vi "RIB - Fuse.vi"(0 "Limits File Path":path, 5 "Results File Path":path, 11 "error in":errorcluster) -> (4 "Results Data Array":string[][](array[string]), 15 "error out":errorcluster)   [LabVIEW 2024]
doc: "Template test"
uses:
  <vilib>/addons/_JKI Toolkits/State Machine/_JKI_lib_State_Machine.llb/Select State(s)_err__jki_lib_state_machine.vi
  <vilib>/addons/_JKI Toolkits/State Machine/_JKI_lib_State_Machine.llb/Select State(s)_bool__jki_lib_state_machine.vi
  <vilib>/addons/_JKI Toolkits/State Machine/_JKI_lib_State_Machine.llb/Periodic Trigger__ogtk__JKI-SM__jki_lib_state_machine.vi
  <userlib>/_OpenG.lib/file/file.llb/Strip Path Extension - String__ogtk.vi
  <vilib>/Utility/file.llb/Read Delimited Spreadsheet (string).vi
  <userlib>/_OpenG.lib/file/file.llb/openg_file.lvlib
  <userlib>/_OpenG.lib/appcontrol/appcontrol.llb/openg_application_control.lvlib
  <userlib>/_OpenG.lib/time/time.llb/openg_time.lvlib
  <vilib>/Utility/file.llb/Write Delimited Spreadsheet (string).vi
panel:
  in  "All Fuses Test":string
  in  "Fuse 9 Test":string
  in  "Fuse 8 Test":string
  in  "Fuse 7 Test":string
  in  "Fuse 6 Test":string
  in  "Fuse 5 Test":string
  in  "Fuse 4 Test":string
  in  "Fuse 3 Test":string
  out "All Fuses Test":bool
  out "Fuse 9 Test":bool
  out "Fuse 8 Test":bool
  out "Fuse 7 Test":bool
  out "Fuse 6 Test":bool
  out "Fuse 5 Test":bool
  out "Fuse 4 Test":bool
  out "Fuse 3 Test":bool
  out "Fuse 2 Test":bool
  out "Fuse 1 Test":bool
  in  "Fuse 2 Test":string
  in  "Fuse 1 Test":string
  in  "connection ID":refnum<k16>
  in  "handle out":u64
  in  "Exit":bool
  # "Fuse Test"
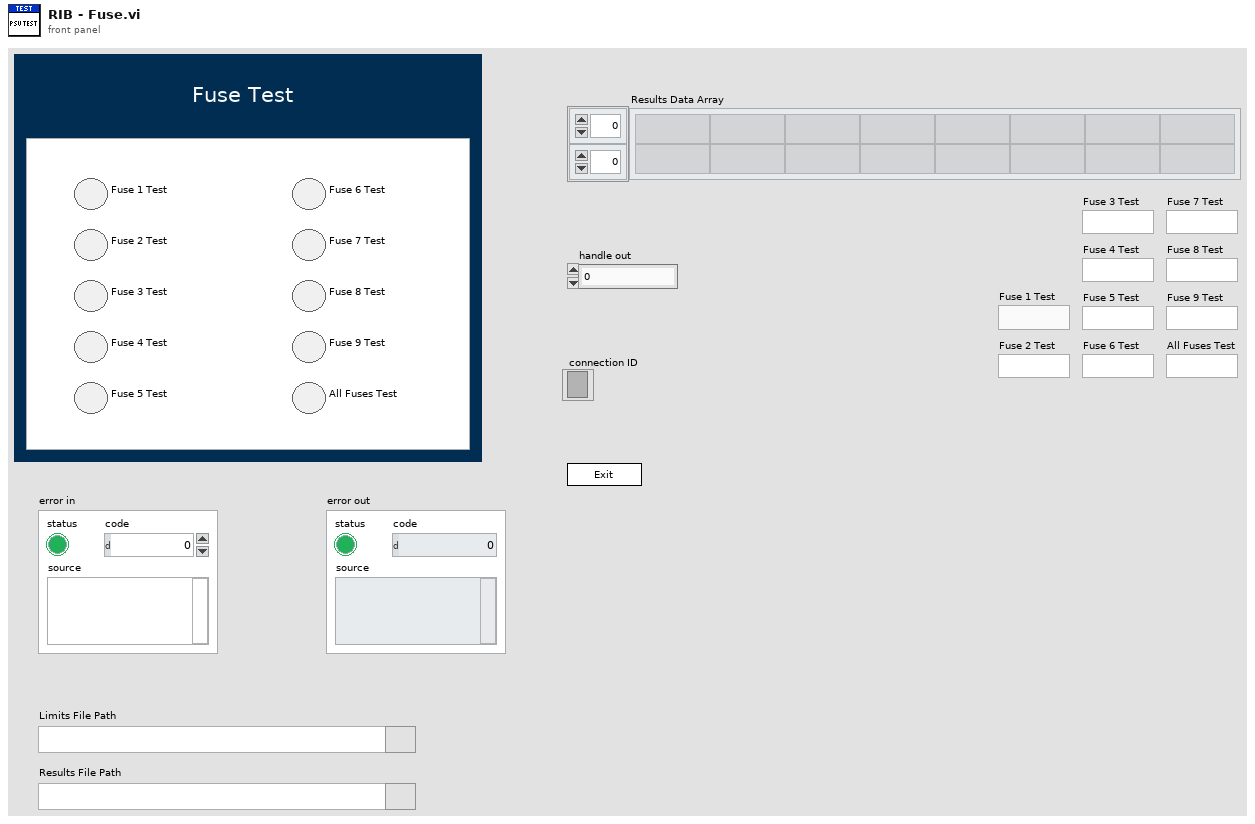
[diagram p1: front panel]
types:
  T1 = enum32{"Invalid", "Standard", "Closed", "Hidden", "Minimized", "Maximized"}
  T2 = enum32{"invalid app kind", "Development System", "Run Time System", "Student Edition", "Embedded LabVIEW", "Evaluation", "Custom"}
  T3 = typedef "FGV - Enum" = enum16{"Cleanup", "Get Data", "Open UDP", "Initialise DAQ", "Initialise I2C"}
  T4 = enum16{"Start Timer", "Get Time", "Pause", "Unpause"}
  T5 = cluster{"Core":cluster{"Current VI Reference":refnum<vi>, "Close Panel on Exit?":bool}, "Limits File Path":path, "Test Limits":string[][], "Results Data Array":string[][], "Results File Path":path, "Voltage":dbl, "connection ID":refnum<k16>, "handle out":u64, "Fuse 1 Test":string, "Fuse 2 Test":string, "Fuse 3 Test":string, "Fuse 4 Test":string, "Fuse 5 Test":string, "Fuse 6 Test":string, "Fuse 7 Test":string, "Fuse 8 Test":string, "Fuse 9 Test":string, "All Fuses Test":string}
  T6 = cluster{"Current VI Reference":refnum<vi>, "Close Panel on Exit?":bool}
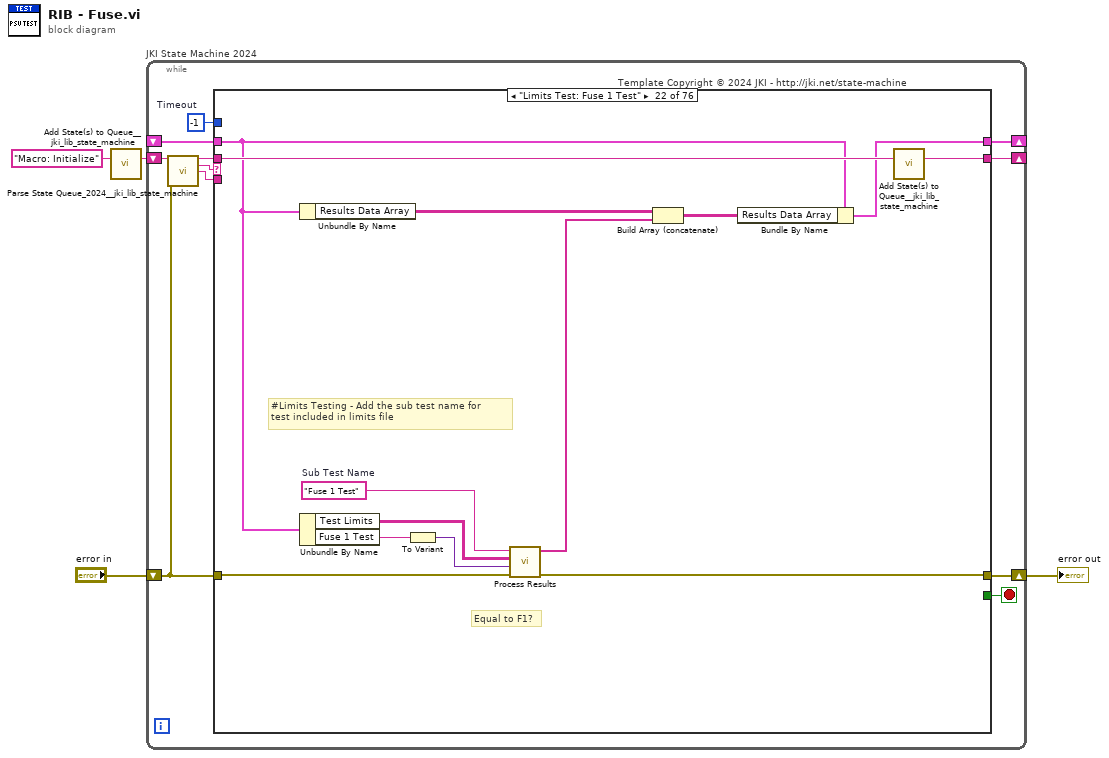
[diagram p0: block diagram]
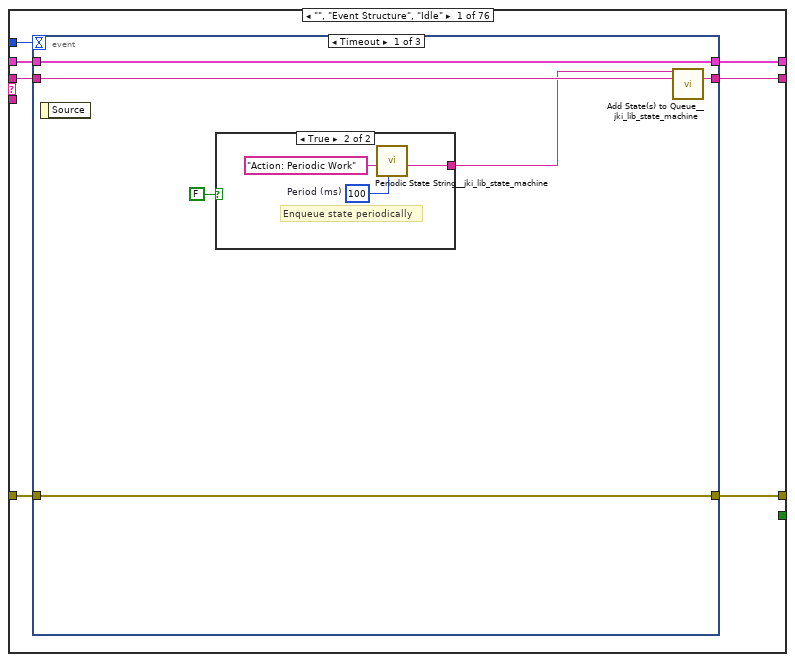
[diagram p2: hidden frame]
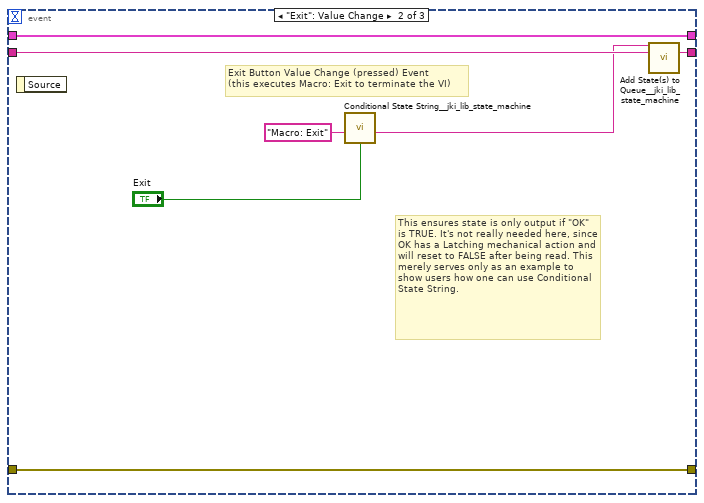
[diagram p4: hidden frame]
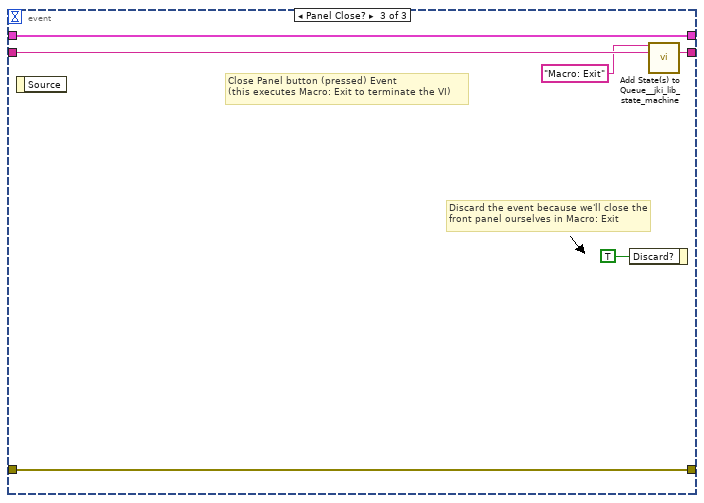
[diagram p5: hidden frame]
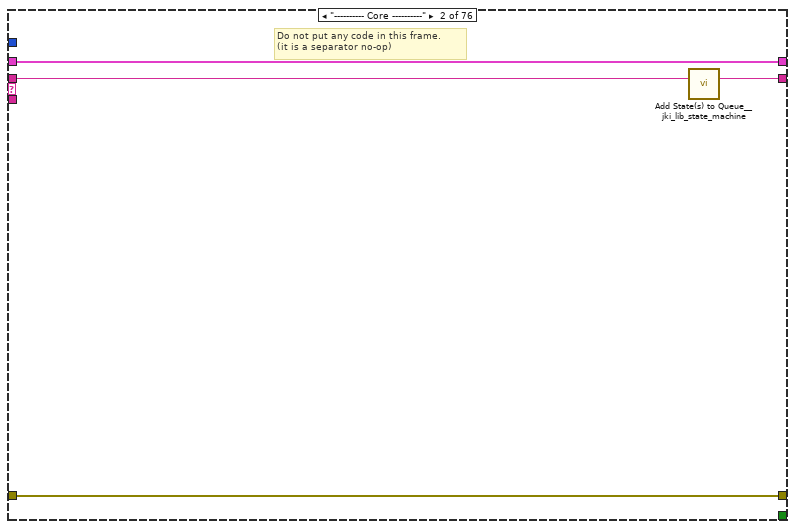
[diagram p6: hidden frame]
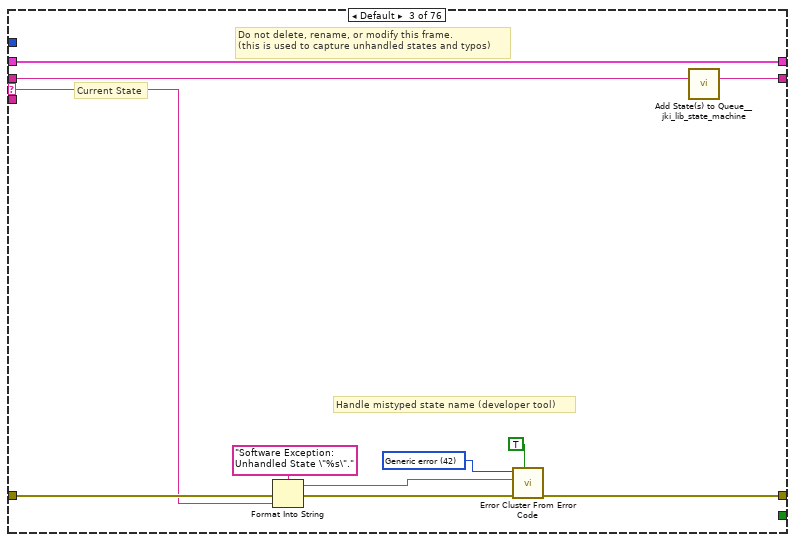
[diagram p7: hidden frame]
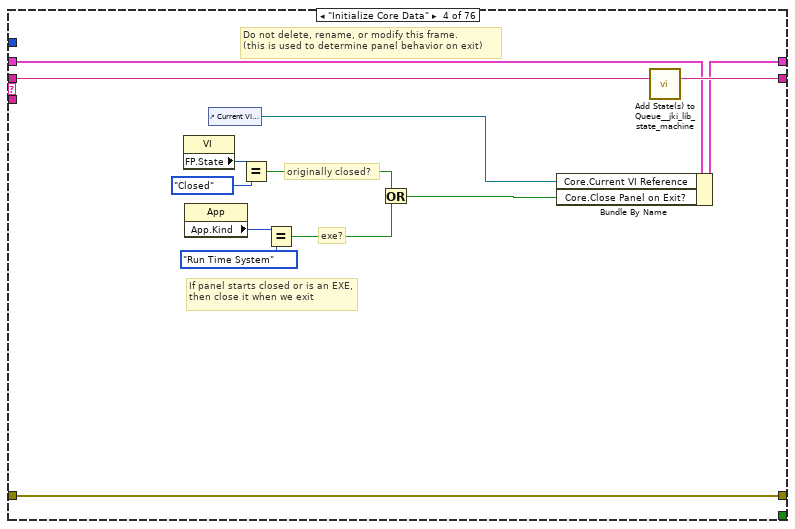
[diagram p8: hidden frame]
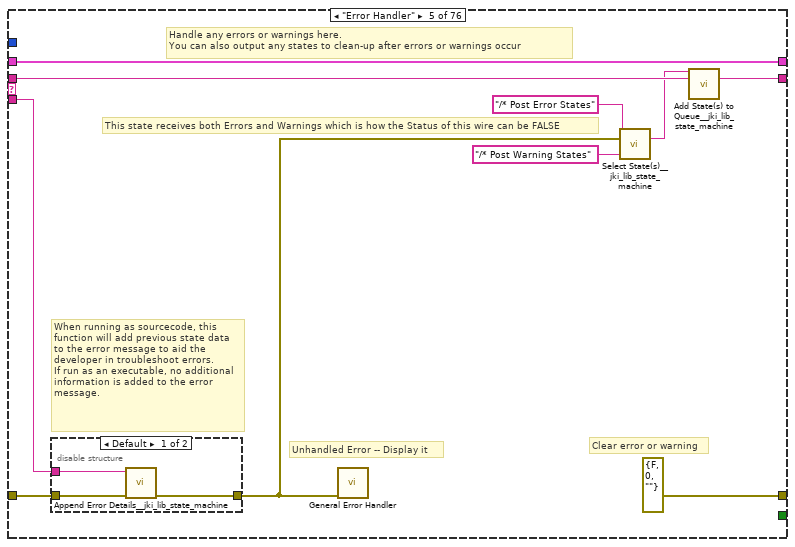
[diagram p9: hidden frame]
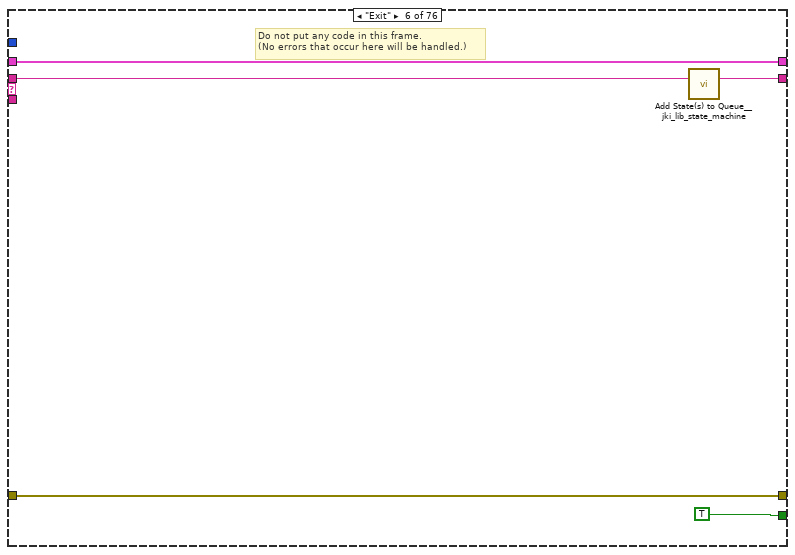
[diagram p11: hidden frame]
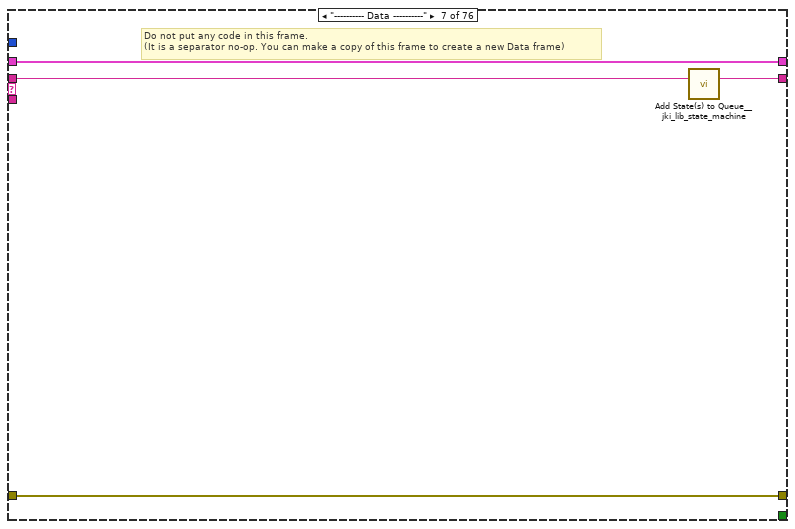
[diagram p12: hidden frame]
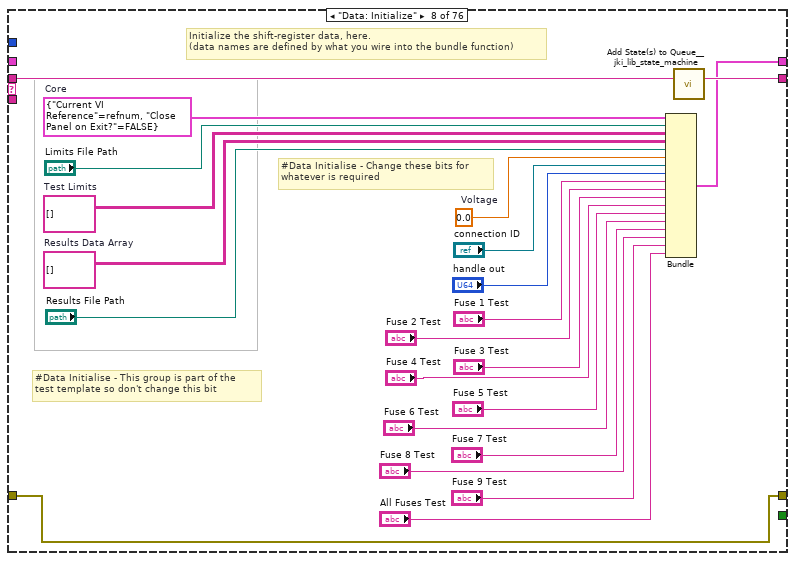
[diagram p13: hidden frame]
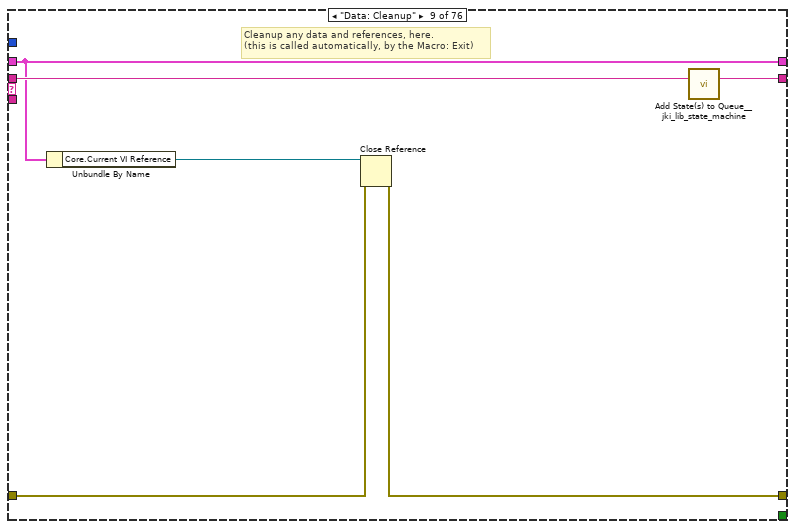
[diagram p14: hidden frame]
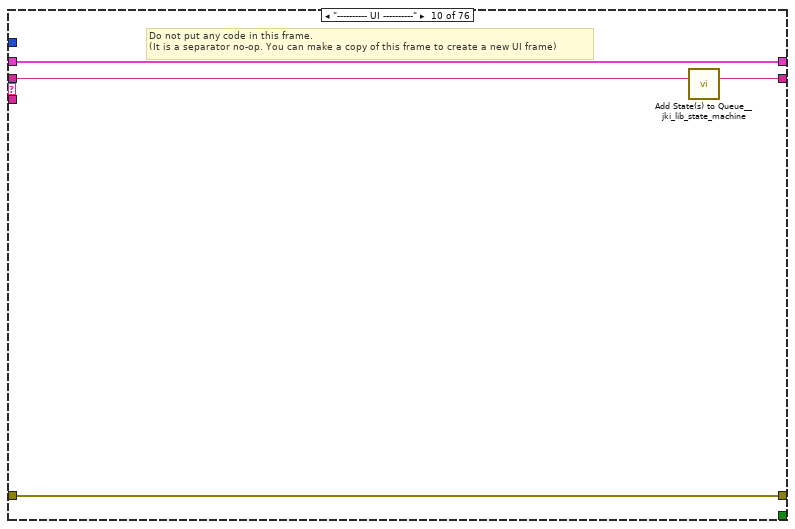
[diagram p15: hidden frame]
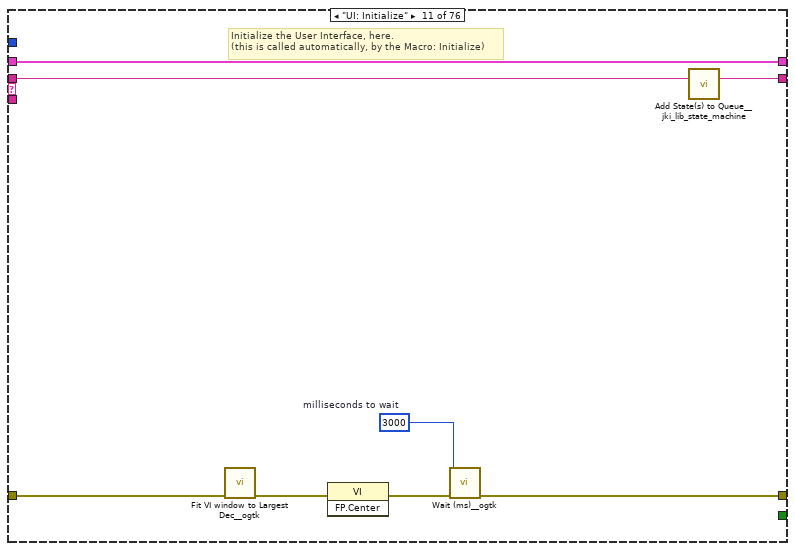
[diagram p16: hidden frame]
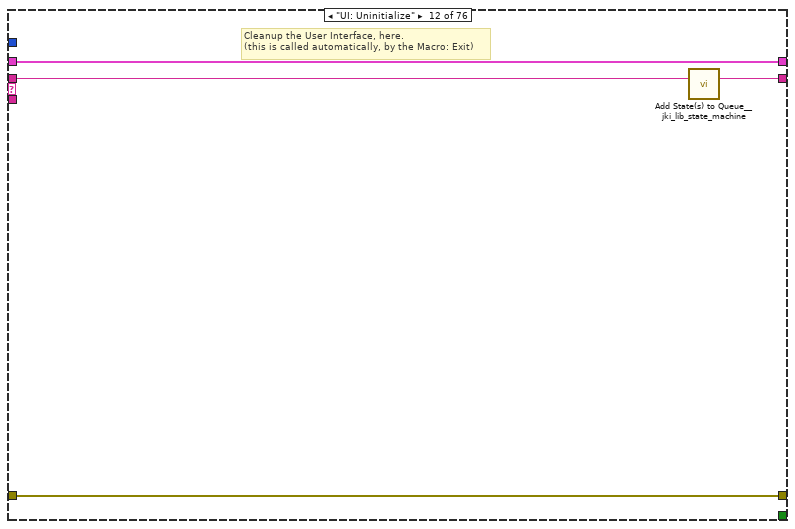
[diagram p17: hidden frame]
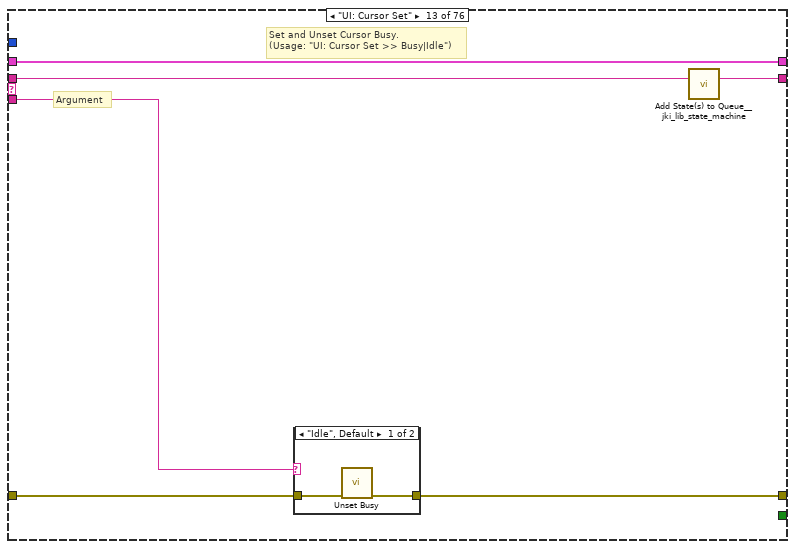
[diagram p18: hidden frame]
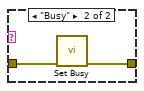
[diagram p19: hidden frame]
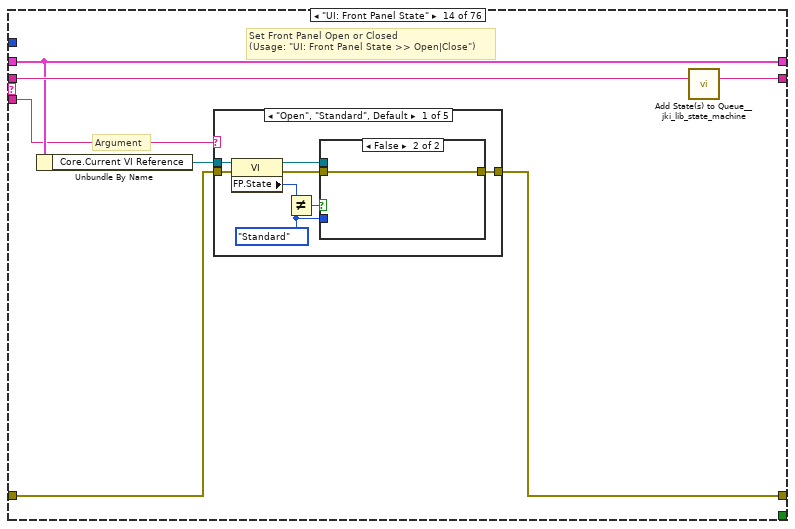
[diagram p20: hidden frame]
diagram:
  n1 = call <vilib>:"Add State(s) to Queue__jki_lib_state_machine.vi"("State(s) in (\"\")"="Macro: Initialize") -> ("States Out"=w4:string)  [unwired: 14 in]
  n2 = while "JKI State Machine 2024" {
    shift-right: [w8] -> _
    shift-left: _ -> [w7]
    shift-right: [w11] -> w1
    shift-left: "error in" -> [w5]
    shift-right: [w10] -> _
    shift-left: w4 -> [w12]
    stop <- w9 stop-if-true
    w6 = -1  # Timeout
    # "Template Copyright © 2024 JKI - http://jki.net/state-machine"
    n3 = call <vilib>:"Parse State Queue_2024__jki_lib_state_machine.vi"("State Queue"=w12, "Error In (no error)"=w5) -> ("Remaining States"=w14:string, "Current State"=w15:string, "Arguments"=w13:string)  [unwired: 11 in]
    n4 = case shown="\"Limits Test: Fuse 1 Test\"" w15 {
      selector: w15 -> [_ _ w49 _ _ _ _ _ _ _ _ _ _ _ _ _ _ _ _ _ _ _ _ _ _ _ _ _ _ _ _ _ _ _ _ _ _ _ _ _ _ _ _ _ _ _ _ _ _ _ _ _ _ _ _ _ _ _ _ _ _ _ _ _ _ _ _ _ _ _ _ _ _ _ _ _]
      tunnel: w14 -> [w22 w48 w53 w72 w82 w91 w95 w117 w123 w127 w135 w139 w145 w156 w225 w230 w235 w240 w249 w253 w266 w283 w296 w309 w322 w335 w348 w361 w374 w387 w400 w404 w413 w417 w426 w432 w442 w468 w479 w486 w496 w522 w533 w540 w550 w576 w587 w594 w604 w630 w641 w648 w658 w684 w695 w702 w712 w738 w749 w756 w766 w792 w803 w810 w820 w846 w857 w864 w874 w900 w911 w918 w928 w954 w965 w974]
      tunnel: w13 -> [_ _ _ _ w77 _ _ _ _ _ _ _ w140 w150 _ _ _ _ _ _ _ _ _ _ _ _ _ _ _ _ _ _ _ _ _ _ _ _ _ _ _ _ _ _ _ _ _ _ _ _ _ _ _ _ _ _ _ _ _ _ _ _ _ _ _ _ _ _ _ _ _ _ _ _ _ _]
      tunnel: w7 -> [w20 w45 w51 w65 w79 w89 w92 _ w118 w124 w133 w137 w143 w152 w222 w227 w232 w237 w247 w250 w256 w275 w288 w301 w314 w327 w340 w353 w366 w379 w392 w401 w409 w414 w424 w430 w440 w448 w477 w484 w494 w502 w531 w538 w548 w556 w585 w592 w602 w610 w639 w646 w656 w664 w693 w700 w710 w718 w747 w754 w764 w772 w801 w808 w818 w826 w855 w862 w872 w880 w909 w916 w926 w934 w963 w972]
      tunnel: [w19 w46 w55 w69 errorcluster {"status"=FALSE, "code"=0, "source"=""} ("error out") w88 w93 w114 w119 w125 w131 w136 w141 w153 w223 w228 w233 w238 w244 w251 w262 w280 w293 w306 w319 w332 w345 w358 w371 w384 w397 w402 w411 w415 w421 w427 w437 w446 w471 w481 w491 w500 w525 w535 w545 w554 w579 w589 w599 w608 w633 w643 w653 w662 w687 w697 w707 w716 w741 w751 w761 w770 w795 w805 w815 w824 w849 w859 w869 w878 w903 w913 w923 w932 w957 w967] -> w11
      tunnel: w5 -> [w16 w46 w54 w69 w78 w88 w93 w114 w120 w125 w132 w136 w142 w154 w223 w228 w233 w238 w244 w251 w261 w279 w292 w305 w318 w331 w344 w357 w370 w383 w396 w402 w410 w415 w422 w428 w436 w449 w472 w482 w490 w503 w526 w536 w544 w557 w580 w590 w598 w611 w634 w644 w652 w665 w688 w698 w706 w719 w742 w752 w760 w773 w796 w806 w814 w827 w850 w860 w868 w881 w904 w914 w922 w935 w958 w966]
      tunnel: [w21 w47 w52 w71 w81 w90 w94 w116 w122 w126 w134 w138 w144 w155 w224 w229 w234 w239 w248 w252 w265 w282 w295 w308 w321 w334 w347 w360 w373 w386 w399 w403 w412 w416 w425 w431 w441 w467 w478 w485 w495 w521 w532 w539 w549 w575 w586 w593 w603 w629 w640 w647 w657 w683 w694 w701 w711 w737 w748 w755 w765 w791 w802 w809 w819 w845 w856 w863 w873 w899 w910 w917 w927 w953 w964 w973] -> w10
      tunnel: [_ _ _ _ _ TRUE _ _ _ _ _ _ _ _ _ _ _ _ _ _ _ _ _ _ _ _ _ _ _ _ _ _ _ _ _ _ _ _ _ _ _ _ _ _ _ _ _ _ _ _ _ _ _ _ _ _ _ _ _ _ _ _ _ _ _ _ _ _ _ _ _ _ _ _ _ _] -> w9
      tunnel: [w18 w45 w51 w70 w79 w89 w92 w115 w118 w124 w133 w137 w143 w152 w222 w227 w232 w237 w247 w250 w255 w274 w287 w300 w313 w326 w339 w352 w365 w378 w391 w401 w409 w414 w423 w430 w439 w466 w477 w484 w493 w520 w531 w538 w547 w574 w585 w592 w601 w628 w639 w646 w655 w682 w693 w700 w709 w736 w747 w754 w763 w790 w801 w808 w817 w844 w855 w862 w871 w898 w909 w916 w925 w952 w963 w971] -> w8
      tunnel: w6 -> [w17 _ _ _ _ _ _ _ _ _ _ _ _ _ _ _ _ _ _ _ _ _ _ _ _ _ _ _ _ _ _ _ _ _ _ _ _ _ _ _ _ _ _ _ _ _ _ _ _ _ _ _ _ _ _ _ _ _ _ _ _ _ _ _ _ _ _ _ _ _ _ _ _ _ _ _]
      frame "", "Event Structure", "Idle" {
        n5 = event shown="[0] Timeout" {
          selector: _ -> [_ _ _]
          dyn-events: _ -> [_ _ _]
          timeout: w17 -> [_ _ _]
          tunnel: w22 -> [w28 w38 w44]
          tunnel: [w27 w37 w43] -> w21
          tunnel: w20 -> [w25 w35 w41]
          tunnel: [w26 w36 w42] -> w19
          tunnel: w16 -> [w26 w36 w42]
          tunnel: [w25 w35 w41] -> w18
          event Timeout {
            n6 = event-data() -> ()  [unwired: 1 in, 1 out]
            n7 = case shown="True" FALSE {
              tunnel: [_ w31] -> w24
              frame False {
              }
              frame True {
                w29 = u32 100  # Period (ms)
                # "Enqueue state periodically"
                n8 = call <vilib>:"Periodic State String__jki_lib_state_machine.vi"("Period (ms)"=w29, "State"="Action: Periodic Work") -> ("State Out"=w31:string)  [unwired: 9 in]
              }
            }
            n9 = call <vilib>:"Add State(s) to Queue__jki_lib_state_machine.vi"("State(s) in Front (\"\")"=w24, "State(s) in (\"\")"=w28) -> ("States Out"=w27:string)  [unwired: 13 in]
          }
          event "Exit": Value Change {
            # "This ensures state is only output if \"OK\" is TRUE. It's not really needed here, since OK has a Latching mechanical action and will reset to FALSE after being read. This merely serves only as an example to show users how one can use Conditional State String."
            # "Exit Button Value Change (pressed) Event\n(this executes Macro: Exit to terminate the VI)"
            n10 = event-data() -> ()  [unwired: 1 in, 1 out]
            n11 = call <vilib>:"Conditional State String__jki_lib_state_machine.vi"("Do State(s)?"="Exit", "State"="Macro: Exit") -> ("State Out"=w32:string)  [unwired: 7 in]
            n12 = call <vilib>:"Add State(s) to Queue__jki_lib_state_machine.vi"("State(s) in Front (\"\")"=w32, "State(s) in (\"\")"=w38) -> ("States Out"=w37:string)  [unwired: 13 in]
          }
          event Panel Close? {
            # "Discard the event because we'll close the front panel ourselves in Macro: Exit"
            # "Close Panel button (pressed) Event\n(this executes Macro: Exit to terminate the VI)"
            n13 = event-data() -> ()  [unwired: 1 in, 1 out]
            n14 = event-data("Discard?"=TRUE) -> ()  [unwired: 1 in, 1 out]
            n15 = call <vilib>:"Add State(s) to Queue__jki_lib_state_machine.vi"("State(s) in Front (\"\")"="Macro: Exit", "State(s) in (\"\")"=w44) -> ("States Out"=w43:string)  [unwired: 13 in]
          }
        }
      }
      frame "---------- Core ----------" {
        # "Do not put any code in this frame.\n(it is a separator no-op)"
        n16 = call <vilib>:"Add State(s) to Queue__jki_lib_state_machine.vi"("State(s) in (\"\")"=w48) -> ("States Out"=w47:string)  [unwired: 14 in]
      }
      frame Default {
        w58 = 42 items=["No error", "Argument error", "Memory is full", "Out of zone", "End of file", "File already open", "Generic file I/O error", "File not found", "File permission error", "Disk is full", "Duplicate path", "Too many files open", "System feature not enabled", "Resource file not found", "Cannot add resource", "Resource not found", "Image not found", "Image memory error", "Pen does not exist", "Config type invalid", "Config token not found", "Config parse error", "Config memory error", "Bad external code format", "Bad external code offset", "External code not present", "Null window", "Destroy window error", "Null menu", "Print aborted", "Bad print record", "Print driver error", "Windows error during printing", "Memory error during printing", "Print dialog error", "Generic print error", "Invalid device refnum", "Device not found", "Device parameter error", "Device unit error", "Cannot open device", "Device call aborted", "Generic error", "Cancelled by user", "Object ID too low", "Object ID too high", "Object not in heap", "Unknown heap", "Unknown object (invalid DefProc)", "Unknown object (DefProc not in table)", "Message out of range", "Invalid (null) method", "Unknown message", "Manager call not supported", "Bad address", "Network operation in progress", "Network operation timed out", "Connection is busy", "Network attribute not supported", "Network error", "Address in use", "System out of memory", "Connection aborted", "Connection refused", "Not connected", "Already connected", "Connection closed", "Initialization error (interapplication manager)", "Bad occurrence", "Wait on unbound occurrence handler", "Occurrence queue overflow", "Datalog type conflict", "Unused", "Unrecognized type (interapplication manager)", "Memory corrupt", "Failed to make temporary DLL", "Old CIN version", "Drag socket not found", "Failed to load drop-object", "Failed to register OLE object", "Failed to release OLE object", "Format specifier type mismatch", "Unknown format specifier", "Too few format specifiers", "Too many format specifiers", "Scan failed", "Newer CIN version", "Error converting to variant", "Runtime menu error", "Password tampered", "Variant attribute not found", "Incompatible variant data type", "Event data is not available", "Event Store is not present", "Occurrence is not found", "Event Queue is not created", "Event info is not available", "Refnum passed is NULL", "Error retrieving Class GUID", "Error retrieving CoClass GUID", "Error retrieving TypeLib GUID.", "Bad built application magic bytes.", "Specific driver is different from the specific driver associated with the Logical Name.", "There is no session opened to the class driver.", "Max Error", "MAX - Error with config objects", "MAX - Error loading configuration", "MAX - Group not supported"]
        # "Current State"
        # "Do not delete, rename, or modify this frame.\n(this is used to capture unhandled states and typos)"
        # "Handle mistyped state name (developer tool)"
        n17 = Format Into String(format string="Software Exception: Unhandled State \"%s\"." ("message"), error in=w54, w49) -> (resulting string=w57:string, error out=w56:errorcluster)  [unwired: 1 in]
        n18 = call <vilib>:"Error Cluster From Error Code.vi"("show call chain? (False)"=TRUE, "error in (no error)"=w56, "error message (\"\")"=w57, "error code (0)"=w58) -> ("error out"=w55:errorcluster)  [unwired: 5 in]
        n19 = call <vilib>:"Add State(s) to Queue__jki_lib_state_machine.vi"("State(s) in (\"\")"=w53) -> ("States Out"=w52:string)  [unwired: 14 in]
      }
      frame "Initialize Core Data" {
        # "Do not delete, rename, or modify this frame.\n(this is used to determine panel behavior on exit)"
        # "originally closed?"
        # "exe?"
        # "If panel starts closed or is an EXE, then close it when we exit"
        n20 = property class="VI"() -> ("FP.State"=w62:T1)  [unwired: 2 in, 2 out]
        n21 = property class="App"() -> ("App.Kind"=w68:T2)  [unwired: 2 in, 2 out]
        n22 = control-ref of="Current VI Reference"() -> (w63:refnum<vi>)
        n23 = Equal?(x=w62, y=T1."Closed" ("Front Panel Window:State")) -> (x = y?=w60:bool)
        n24 = Equal?(x=w68, y=T2."Run Time System" ("Application:Kind")) -> (x = y?=w66:bool)
        n25 = Or(x=w60, y=w66) -> (x .or. y?=w64:bool)
        n26 = Bundle By Name(cluster=w65, "Core.Current VI Reference"=w63, "Core.Close Panel on Exit?"=w64) -> (w70:T5)
        n27 = call <vilib>:"Add State(s) to Queue__jki_lib_state_machine.vi"("State(s) in (\"\")"=w72) -> ("States Out"=w71:string)  [unwired: 14 in]
      }
      frame "Error Handler" {
        # "When running as sourcecode, this function will add previous state data to the error message to aid the developer in troubleshoot errors.\nIf run as an executable, no additional information is added to the error message."
        # "This state receives both Errors and Warnings which is how the Status of this wire can be FALSE"
        # "Unhandled Error -- Display it"
        # "Handle any errors or warnings here.\nYou can also output any states to clean-up after errors or warnings occur"
        # "Clear error or warning"
        n28 = disable-structure shown="Default" {
          disable-tunnel: w78 -> [w85 w86]
          disable-tunnel: w77 -> [w84 _]
          disable-tunnel: [w83 w86] -> w76
          frame condition #0 (active) {
            n29 = call <vilib>:"Append Error Details__jki_lib_state_machine.vi"("error in (no error)"=w85, "Previous State and Argument(s)"=w84) -> ("error out"=w83:errorcluster)  [unwired: 9 in]
          }
          frame condition #1 {
          }
        }
        n30 = call <vilib>:"General Error Handler.vi"("error in (no error)"=w76) -> ()  [unwired: 10 in, 5 out]
        n31 = call-poly <vilib>:"Select State(s)__jki_lib_state_machine.vi"("State(s) if True (\"\")"="/* Post Error States", "Select"=w76, "State(s) if False (\"\")"="/* Post Warning States") -> ("States Out"=w74:string)  [unwired: 12 in]
        n32 = call <vilib>:"Add State(s) to Queue__jki_lib_state_machine.vi"("State(s) in Front (\"\")"=w74, "State(s) in (\"\")"=w82) -> ("States Out"=w81:string)  [unwired: 13 in]
      }
      frame "Exit" {
        # "Do not put any code in this frame.\n(No errors that occur here will be handled.)"
        n33 = call <vilib>:"Add State(s) to Queue__jki_lib_state_machine.vi"("State(s) in (\"\")"=w91) -> ("States Out"=w90:string)  [unwired: 14 in]
      }
      frame "---------- Data ----------" {
        # "Do not put any code in this frame.\n(It is a separator no-op. You can make a copy of this frame to create a new Data frame)"
        n34 = call <vilib>:"Add State(s) to Queue__jki_lib_state_machine.vi"("State(s) in (\"\")"=w95) -> ("States Out"=w94:string)  [unwired: 14 in]
      }
      frame "Data: Initialize" {
        w108 = 0.0  # Voltage
        w110 = string[][] []  # Results Data Array
        w111 = string[][] []  # Test Limits
        w113 = T6 {"Current VI Reference"=refnum, "Close Panel on Exit?"=FALSE}  # Core
        # "#Data Initialise - Change these bits for\nwhatever is required"
        # "#Data Initialise - This group is part of the\ntest template so don't change this bit"
        # "Initialize the shift-register data, here.\n(data names are defined by what you wire into the bundle function)"
        n35 = Bundle("Core"=w113, "Limits File Path"="Limits File Path", "Test Limits"=w111, "Results Data Array"=w110, "Results File Path"="Results File Path", "Voltage"=w108, "connection ID"="connection ID", "handle out"="handle out", "Fuse 1 Test"="Fuse 1 Test", "Fuse 2 Test"="Fuse 2 Test", "Fuse 3 Test"="Fuse 3 Test", "Fuse 4 Test"="Fuse 4 Test", "Fuse 5 Test"="Fuse 5 Test", "Fuse 6 Test"="Fuse 6 Test", "Fuse 7 Test"="Fuse 7 Test", "Fuse 8 Test"="Fuse 8 Test", "Fuse 9 Test"="Fuse 9 Test", "All Fuses Test"="All Fuses Test") -> (w115:T5)  [unwired: 1 in]
        n36 = call <vilib>:"Add State(s) to Queue__jki_lib_state_machine.vi"("State(s) in (\"\")"=w117) -> ("States Out"=w116:string)  [unwired: 14 in]
      }
      frame "Data: Cleanup" {
        # "Cleanup any data and references, here.\n(this is called automatically, by the Macro: Exit)"
        n37 = Unbundle By Name(w118) -> ("Core.Current VI Reference"=w121:refnum<vi>)
        n38 = Close Reference(reference=w121, error in (no error)=w120) -> (error out=w119:errorcluster)
        n39 = call <vilib>:"Add State(s) to Queue__jki_lib_state_machine.vi"("State(s) in (\"\")"=w123) -> ("States Out"=w122:string)  [unwired: 14 in]
      }
      frame "---------- UI ----------" {
        # "Do not put any code in this frame.\n(It is a separator no-op. You can make a copy of this frame to create a new UI frame)"
        n40 = call <vilib>:"Add State(s) to Queue__jki_lib_state_machine.vi"("State(s) in (\"\")"=w127) -> ("States Out"=w126:string)  [unwired: 14 in]
      }
      frame "UI: Initialize" {
        w130 = u32 3000  # milliseconds to wait
        # "Initialize the User Interface, here.\n(this is called automatically, by the Macro: Initialize)"
        n41 = call <userlib>:"Fit VI window to Largest Dec__ogtk.vi"("error in (no error)"=w132) -> ("error out"=w128:errorcluster)  [unwired: 5 in, 1 out]
        n42 = invoke class="VI" method="FP.Center"(error in=w128) -> (error out=w129:errorcluster)  [unwired: 2 in, 2 out]
        n43 = call <userlib>:"Wait (ms)__ogtk.vi"("error in (no error)"=w129, "milliseconds to wait"=w130) -> ("error out"=w131:errorcluster)  [unwired: 8 in, 1 out]
        n44 = call <vilib>:"Add State(s) to Queue__jki_lib_state_machine.vi"("State(s) in (\"\")"=w135) -> ("States Out"=w134:string)  [unwired: 14 in]
      }
      frame "UI: Uninitialize" {
        # "Cleanup the User Interface, here.\n(this is called automatically, by the Macro: Exit)"
        n45 = call <vilib>:"Add State(s) to Queue__jki_lib_state_machine.vi"("State(s) in (\"\")"=w139) -> ("States Out"=w138:string)  [unwired: 14 in]
      }
      frame "UI: Cursor Set" {
        # "Argument"
        # "Set and Unset Cursor Busy.\n(Usage: \"UI: Cursor Set >> Busy|Idle\")"
        n46 = case shown="\"Idle\", Default" w140 {
          tunnel: w142 -> [w147 w149]
          tunnel: [w146 w148] -> w141
          frame "Idle", Default {
            n47 = call <vilib>:"Unset Busy.vi"("error in (no error)"=w147) -> ("error out"=w146:errorcluster)  [unwired: 10 in]
          }
          frame "Busy" {
            n48 = call <vilib>:"Set Busy.vi"("error in (no error)"=w149) -> ("error out"=w148:errorcluster)  [unwired: 9 in, 1 out]
          }
        }
        n49 = call <vilib>:"Add State(s) to Queue__jki_lib_state_machine.vi"("State(s) in (\"\")"=w145) -> ("States Out"=w144:string)  [unwired: 14 in]
      }
      frame "UI: Front Panel State" {
        # "Argument"
        # "Set Front Panel Open or Closed\n(Usage: \"UI: Front Panel State >> Open|Close\")"
        n50 = Unbundle By Name(w152) -> ("Core.Current VI Reference"=w151:refnum<vi>)
        n51 = case shown="\"Open\", \"Standard\", Default" w150 {
          tunnel: w154 -> [w162 w177 w188 w201 w214]
          tunnel: [w164 w178 w190 w203 w216] -> w153
          tunnel: w151 -> [w163 w175 w189 w202 w215]
          frame "Open", "Standard", Default {
            w157 = T1."Standard" ("State")
            n52 = property class="VI"(reference=w163, error in=w162) -> (reference out=w160:refnum<vi>, error out=w161:errorcluster, "FP.State"=w159:T1)
            n53 = Not Equal?(x=w159, y=w157) -> (x != y?=w158:bool)
            n54 = case shown="False" w158 {
              tunnel: [w168 w170] -> w164
              tunnel: w161 -> [w167 w170]
              tunnel: w160 -> [w166 _]
              tunnel: w157 -> [w165 _]
              frame True {
                n55 = invoke class="VI" method="FP.Open"(reference=w166, error in=w167, "Activate"=TRUE, "State"=w165) -> (error out=w168:errorcluster)  [unwired: 1 in, 4 out]
              }
              frame False {
              }
            }
          }
          frame "Close", "Closed" {
            n56 = property class="VI"(reference=w175, error in=w177) -> (reference out=w174:refnum<vi>, error out=w176:errorcluster, "FP.State"=w172:T1)
            n57 = Not Equal?(x=w172, y=T1."Closed" ("Front Panel Window:State")) -> (x != y?=w171:bool)
            n58 = case shown="True" w171 {
              tunnel: [w179 w182] -> w178
              tunnel: w176 -> [w179 w181]
              tunnel: w174 -> [_ w180]
              frame False {
              }
              frame True {
                n59 = invoke class="VI" method="FP.Close"(reference=w180, error in=w181) -> (error out=w182:errorcluster)  [unwired: 1 in, 2 out]
              }
            }
          }
          frame "Hidden", "Hide" {
            w183 = T1."Hidden" ("State")
            n60 = property class="VI"(reference=w189, error in=w188) -> (reference out=w186:refnum<vi>, error out=w187:errorcluster, "FP.State"=w185:T1)
            n61 = Not Equal?(x=w185, y=w183) -> (x != y?=w184:bool)
            n62 = case shown="True" w184 {
              tunnel: [w194 w195] -> w190
              tunnel: w187 -> [w193 w195]
              tunnel: w186 -> [w192 _]
              tunnel: w183 -> [w191 _]
              frame True {
                n63 = invoke class="VI" method="FP.Open"(reference=w192, error in=w193, "State"=w191) -> (error out=w194:errorcluster)  [unwired: 2 in, 4 out]
              }
              frame False {
              }
            }
          }
          frame "Minimize", "Minimized" {
            w196 = T1."Minimized" ("State")
            n64 = property class="VI"(reference=w202, error in=w201) -> (reference out=w199:refnum<vi>, error out=w200:errorcluster, "FP.State"=w198:T1)
            n65 = Not Equal?(x=w198, y=w196) -> (x != y?=w197:bool)
            n66 = case shown="True" w197 {
              tunnel: [w207 w208] -> w203
              tunnel: w200 -> [w206 w208]
              tunnel: w199 -> [w205 _]
              tunnel: w196 -> [w204 _]
              frame True {
                n67 = invoke class="VI" method="FP.Open"(reference=w205, error in=w206, "State"=w204) -> (error out=w207:errorcluster)  [unwired: 2 in, 4 out]
              }
              frame False {
              }
            }
          }
          frame "Maximize", "Maximized" {
            w209 = T1."Maximized" ("State")
            n68 = property class="VI"(reference=w215, error in=w214) -> (reference out=w212:refnum<vi>, error out=w213:errorcluster, "FP.State"=w211:T1)
            n69 = Not Equal?(x=w211, y=w209) -> (x != y?=w210:bool)
            n70 = case shown="True" w210 {
              tunnel: [w220 w221] -> w216
              tunnel: w213 -> [w219 w221]
              tunnel: w212 -> [w218 _]
              tunnel: w209 -> [w217 _]
              frame True {
                n71 = invoke class="VI" method="FP.Open"(reference=w218, error in=w219, "State"=w217) -> (error out=w220:errorcluster)  [unwired: 2 in, 4 out]
              }
              frame False {
              }
            }
          }
        }
        n72 = call <vilib>:"Add State(s) to Queue__jki_lib_state_machine.vi"("State(s) in (\"\")"=w156) -> ("States Out"=w155:string)  [unwired: 14 in]
      }
      frame "---------- Macro ----------" {
        # "Do not put any code in this frame.\n(It is a separator no-op. You can make a copy of this frame to create a new Macro frame)"
        n73 = call <vilib>:"Add State(s) to Queue__jki_lib_state_machine.vi"("State(s) in (\"\")"=w225) -> ("States Out"=w224:string)  [unwired: 14 in]
      }
      frame "Macro: Initialize" {
        # "Initialization Macro\n(This is called once, when the VI starts)"
        n74 = call <vilib>:"Add State(s) to Queue__jki_lib_state_machine.vi"("State(s) in Front (\"\")"="Data: Initialize\nInitialize Core Data\nUI: Initialize\nUI: Front Panel State >> Open\nFuse Test: Initialise\nMacro: Test", "State(s) in (\"\")"=w230) -> ("States Out"=w229:string)  [unwired: 13 in]
      }
      frame "Macro: Test" {
        # "#Test Macro - Add the sequence \nfor measurments and limits testing here"
        n75 = call <vilib>:"Add State(s) to Queue__jki_lib_state_machine.vi"("State(s) in Front (\"\")"="Limits Test: Read Limits File\nFuse Test: F1 Start Timer\nFuse Test: F1 I2C Measurment", "State(s) in (\"\")"=w235) -> ("States Out"=w234:string)  [unwired: 13 in]
      }
      frame "Macro: Limits" {
        # "Do not put any code in this frame.\n(It is a separator no-op. You can make a copy of this frame to create a new Macro frame)"
        n76 = call <vilib>:"Add State(s) to Queue__jki_lib_state_machine.vi"("State(s) in Front (\"\")"="Limits Test: Fuse 1 Test\nLimits Test: Fuse 2 Test\nLimits Test: Fuse 3 Test\nLimits Test: Fuse 4 Test\nLimits Test: Fuse 5 Test\nLimits Test: Fuse 6 Test\nLimits Test: Fuse 7 Test\nLimits Test: Fuse 8 Test\nLimits Test: Fuse 9 Test\nLimits Test: All Fuses Test\nResults Data: Write Results Data\nMacro: Exit", "State(s) in (\"\")"=w240) -> ("States Out"=w239:string)  [unwired: 13 in]
      }
      frame "Macro: Exit" {
        # "Exit Macro\n(This is called once, when the VI exits)"
        n77 = Unbundle By Name(w247) -> ("Core.Close Panel on Exit?"=w242:bool)
        n78 = call <vilib>:"Conditional State String__jki_lib_state_machine.vi"("Do State(s)?"=w242, "State"="UI: Front Panel State >> Close") -> ("State Out"=w241:string)  [unwired: 7 in]
        n79 = call <vilib>:"Add State(s) to Queue__jki_lib_state_machine.vi"("State(s) in (\"\")"=w241, "State(s) at Back (\"\")"="Fuse Test: Cleanup\nUI: Uninitialize\nData: Cleanup\nExit") -> ("States Out"=w245:string)  [unwired: 13 in]
        n80 = call <vilib>:"Add State(s) to Queue__jki_lib_state_machine.vi"("State(s) in Front (\"\")"=w245, "State(s) in (\"\")"=w249) -> ("States Out"=w248:string)  [unwired: 13 in]
      }
      frame "---------- Limits Test ----------" {
        # "Template Separator\n(You can make a copy of, or modify, this frame)"
        n81 = call <vilib>:"Add State(s) to Queue__jki_lib_state_machine.vi"("State(s) in (\"\")"=w253) -> ("States Out"=w252:string)  [unwired: 14 in]
      }
      frame "Limits Test: Read Limits File" {
        w259 = ","  # delimiter (\t)
        n82 = Unbundle By Name(w256) -> ("Limits File Path"=w260:path)
        n83 = Current VI's Path "Test Case Path"() -> (path=w264:path)
        n84 = call-poly <vilib>:"Read Delimited Spreadsheet.vi"("file path (dialog if empty)"=w260, "error in (no error)"=w261, "delimiter (\\t)"=w259) -> ("all rows"=w257:string[][], "error out"=w262:errorcluster)  [unwired: 7 in, 4 out]
        n85 = Strip Path(path=w264) -> (name=w263:string)  [unwired: 1 out]
        n86 = call-poly <userlib>:"Strip Path Extension__ogtk.vi"("path"=w263) -> ("root"=w258:string)  [unwired: 1 out]
        n87 = for {
          tunnel: w258 -> [w270]
          tunnel: w257 -> [w268] mode=indexing
          tunnel: [w268] -> w254 mode=indexing if=w267
          n88 = Index Array(array=w268) -> (element=w269:string)  [unwired: 1 in]
          n89 = Equal?(x=w270, y=w269) -> (x = y?=w267:bool)
        }
        n90 = Bundle By Name(cluster=w256, "Test Limits"=w254) -> (w255:T5)
        n91 = call <vilib>:"Add State(s) to Queue__jki_lib_state_machine.vi"("State(s) in (\"\")"=w266) -> ("States Out"=w265:string)  [unwired: 14 in]
      }
      frame "Limits Test: Fuse 1 Test" {
        w276 = "Fuse 1 Test"  # Sub Test Name
        # "Equal to F1?"
        # "#Limits Testing - Add the sub test name for\ntest included in limits file"
        n92 = Unbundle By Name(w275) -> ("Results Data Array"=w273:string[][])
        n93 = Unbundle By Name(w275) -> ("Test Limits"=w277:string[][], "Fuse 1 Test"=w281:string)
        n94 = To Variant(anything=w281) -> (Variant=w278:variant)
        n95 = call "Process Results.vi"("error in (no error)"=w279, "Measurment"=w278, "Test Limits"=w277, "Sub Test Name"=w276) -> ("error out"=w280:errorcluster, "Results Data"=w272:string[])  [unwired: 6 in]
        n96 = Build Array (concatenate)(w273, w272) -> (w271:string[][])
        n97 = Bundle By Name(cluster=w275, "Results Data Array"=w271) -> (w274:T5)
        n98 = call <vilib>:"Add State(s) to Queue__jki_lib_state_machine.vi"("State(s) in (\"\")"=w283) -> ("States Out"=w282:string)  [unwired: 14 in]
      }
      frame "Limits Test: Fuse 2 Test" {
        w289 = "Fuse 2 Test"  # Sub Test Name
        # "Equal to F1?"
        # "#Limits Testing - Add the sub test name for\ntest included in limits file"
        n99 = Unbundle By Name(w288) -> ("Results Data Array"=w286:string[][])
        n100 = Unbundle By Name(w288) -> ("Test Limits"=w290:string[][], "Fuse 2 Test"=w294:string)
        n101 = To Variant(anything=w294) -> (Variant=w291:variant)
        n102 = call "Process Results.vi"("error in (no error)"=w292, "Measurment"=w291, "Test Limits"=w290, "Sub Test Name"=w289) -> ("error out"=w293:errorcluster, "Results Data"=w285:string[])  [unwired: 6 in]
        n103 = Build Array (concatenate)(w286, w285) -> (w284:string[][])
        n104 = Bundle By Name(cluster=w288, "Results Data Array"=w284) -> (w287:T5)
        n105 = call <vilib>:"Add State(s) to Queue__jki_lib_state_machine.vi"("State(s) in (\"\")"=w296) -> ("States Out"=w295:string)  [unwired: 14 in]
      }
      frame "Limits Test: Fuse 3 Test" {
        w302 = "Fuse 3 Test"  # Sub Test Name
        # "Equal to F1?"
        # "#Limits Testing - Add the sub test name for\ntest included in limits file"
        n106 = Unbundle By Name(w301) -> ("Results Data Array"=w299:string[][])
        n107 = Unbundle By Name(w301) -> ("Test Limits"=w303:string[][], "Fuse 3 Test"=w307:string)
        n108 = To Variant(anything=w307) -> (Variant=w304:variant)
        n109 = call "Process Results.vi"("error in (no error)"=w305, "Measurment"=w304, "Test Limits"=w303, "Sub Test Name"=w302) -> ("error out"=w306:errorcluster, "Results Data"=w298:string[])  [unwired: 6 in]
        n110 = Build Array (concatenate)(w299, w298) -> (w297:string[][])
        n111 = Bundle By Name(cluster=w301, "Results Data Array"=w297) -> (w300:T5)
        n112 = call <vilib>:"Add State(s) to Queue__jki_lib_state_machine.vi"("State(s) in (\"\")"=w309) -> ("States Out"=w308:string)  [unwired: 14 in]
      }
      frame "Limits Test: Fuse 4 Test" {
        w315 = "Fuse 4 Test"  # Sub Test Name
        # "Equal to F1?"
        # "#Limits Testing - Add the sub test name for\ntest included in limits file"
        n113 = Unbundle By Name(w314) -> ("Results Data Array"=w312:string[][])
        n114 = Unbundle By Name(w314) -> ("Test Limits"=w316:string[][], "Fuse 4 Test"=w320:string)
        n115 = To Variant(anything=w320) -> (Variant=w317:variant)
        n116 = call "Process Results.vi"("error in (no error)"=w318, "Measurment"=w317, "Test Limits"=w316, "Sub Test Name"=w315) -> ("error out"=w319:errorcluster, "Results Data"=w311:string[])  [unwired: 6 in]
        n117 = Build Array (concatenate)(w312, w311) -> (w310:string[][])
        n118 = Bundle By Name(cluster=w314, "Results Data Array"=w310) -> (w313:T5)
        n119 = call <vilib>:"Add State(s) to Queue__jki_lib_state_machine.vi"("State(s) in (\"\")"=w322) -> ("States Out"=w321:string)  [unwired: 14 in]
      }
      frame "Limits Test: Fuse 5 Test" {
        w328 = "Fuse 5 Test"  # Sub Test Name
        # "Equal to F1?"
        # "#Limits Testing - Add the sub test name for\ntest included in limits file"
        n120 = Unbundle By Name(w327) -> ("Results Data Array"=w325:string[][])
        n121 = Unbundle By Name(w327) -> ("Test Limits"=w329:string[][], "Fuse 5 Test"=w333:string)
        n122 = To Variant(anything=w333) -> (Variant=w330:variant)
        n123 = call "Process Results.vi"("error in (no error)"=w331, "Measurment"=w330, "Test Limits"=w329, "Sub Test Name"=w328) -> ("error out"=w332:errorcluster, "Results Data"=w324:string[])  [unwired: 6 in]
        n124 = Build Array (concatenate)(w325, w324) -> (w323:string[][])
        n125 = Bundle By Name(cluster=w327, "Results Data Array"=w323) -> (w326:T5)
        n126 = call <vilib>:"Add State(s) to Queue__jki_lib_state_machine.vi"("State(s) in (\"\")"=w335) -> ("States Out"=w334:string)  [unwired: 14 in]
      }
      frame "Limits Test: Fuse 6 Test" {
        w341 = "Fuse 6 Test"  # Sub Test Name
        # "Equal to F1?"
        # "#Limits Testing - Add the sub test name for\ntest included in limits file"
        n127 = Unbundle By Name(w340) -> ("Results Data Array"=w338:string[][])
        n128 = Unbundle By Name(w340) -> ("Test Limits"=w342:string[][], "Fuse 6 Test"=w346:string)
        n129 = To Variant(anything=w346) -> (Variant=w343:variant)
        n130 = call "Process Results.vi"("error in (no error)"=w344, "Measurment"=w343, "Test Limits"=w342, "Sub Test Name"=w341) -> ("error out"=w345:errorcluster, "Results Data"=w337:string[])  [unwired: 6 in]
        n131 = Build Array (concatenate)(w338, w337) -> (w336:string[][])
        n132 = Bundle By Name(cluster=w340, "Results Data Array"=w336) -> (w339:T5)
        n133 = call <vilib>:"Add State(s) to Queue__jki_lib_state_machine.vi"("State(s) in (\"\")"=w348) -> ("States Out"=w347:string)  [unwired: 14 in]
      }
      frame "Limits Test: Fuse 7 Test" {
        w354 = "Fuse 7 Test"  # Sub Test Name
        # "Equal to F1?"
        # "#Limits Testing - Add the sub test name for\ntest included in limits file"
        n134 = Unbundle By Name(w353) -> ("Results Data Array"=w351:string[][])
        n135 = Unbundle By Name(w353) -> ("Test Limits"=w355:string[][], "Fuse 7 Test"=w359:string)
        n136 = To Variant(anything=w359) -> (Variant=w356:variant)
        n137 = call "Process Results.vi"("error in (no error)"=w357, "Measurment"=w356, "Test Limits"=w355, "Sub Test Name"=w354) -> ("error out"=w358:errorcluster, "Results Data"=w350:string[])  [unwired: 6 in]
        n138 = Build Array (concatenate)(w351, w350) -> (w349:string[][])
        n139 = Bundle By Name(cluster=w353, "Results Data Array"=w349) -> (w352:T5)
        n140 = call <vilib>:"Add State(s) to Queue__jki_lib_state_machine.vi"("State(s) in (\"\")"=w361) -> ("States Out"=w360:string)  [unwired: 14 in]
      }
      frame "Limits Test: Fuse 8 Test" {
        w367 = "Fuse 8 Test"  # Sub Test Name
        # "Equal to F1?"
        # "#Limits Testing - Add the sub test name for\ntest included in limits file"
        n141 = Unbundle By Name(w366) -> ("Results Data Array"=w364:string[][])
        n142 = Unbundle By Name(w366) -> ("Test Limits"=w368:string[][], "Fuse 8 Test"=w372:string)
        n143 = To Variant(anything=w372) -> (Variant=w369:variant)
        n144 = call "Process Results.vi"("error in (no error)"=w370, "Measurment"=w369, "Test Limits"=w368, "Sub Test Name"=w367) -> ("error out"=w371:errorcluster, "Results Data"=w363:string[])  [unwired: 6 in]
        n145 = Build Array (concatenate)(w364, w363) -> (w362:string[][])
        n146 = Bundle By Name(cluster=w366, "Results Data Array"=w362) -> (w365:T5)
        n147 = call <vilib>:"Add State(s) to Queue__jki_lib_state_machine.vi"("State(s) in (\"\")"=w374) -> ("States Out"=w373:string)  [unwired: 14 in]
      }
      frame "Limits Test: Fuse 9 Test" {
        w380 = "Fuse 9 Test"  # Sub Test Name
        # "Equal to F1?"
        # "#Limits Testing - Add the sub test name for\ntest included in limits file"
        n148 = Unbundle By Name(w379) -> ("Results Data Array"=w377:string[][])
        n149 = Unbundle By Name(w379) -> ("Test Limits"=w381:string[][], "Fuse 9 Test"=w385:string)
        n150 = To Variant(anything=w385) -> (Variant=w382:variant)
        n151 = call "Process Results.vi"("error in (no error)"=w383, "Measurment"=w382, "Test Limits"=w381, "Sub Test Name"=w380) -> ("error out"=w384:errorcluster, "Results Data"=w376:string[])  [unwired: 6 in]
        n152 = Build Array (concatenate)(w377, w376) -> (w375:string[][])
        n153 = Bundle By Name(cluster=w379, "Results Data Array"=w375) -> (w378:T5)
        n154 = call <vilib>:"Add State(s) to Queue__jki_lib_state_machine.vi"("State(s) in (\"\")"=w387) -> ("States Out"=w386:string)  [unwired: 14 in]
      }
      frame "Limits Test: All Fuses Test" {
        w393 = "All Fuses Test"  # Sub Test Name
        # "Equal to F1?"
        # "#Limits Testing - Add the sub test name for\ntest included in limits file"
        n155 = Unbundle By Name(w392) -> ("Test Limits"=w394:string[][], "All Fuses Test"=w398:string)
        n156 = Unbundle By Name(w392) -> ("Results Data Array"=w390:string[][])
        n157 = To Variant(anything=w398) -> (Variant=w395:variant)
        n158 = call "Process Results.vi"("error in (no error)"=w396, "Measurment"=w395, "Test Limits"=w394, "Sub Test Name"=w393) -> ("error out"=w397:errorcluster, "Results Data"=w389:string[])  [unwired: 6 in]
        n159 = Build Array (concatenate)(w390, w389) -> (w388:string[][])
        n160 = Bundle By Name(cluster=w392, "Results Data Array"=w388) -> (w391:T5)
        n161 = call <vilib>:"Add State(s) to Queue__jki_lib_state_machine.vi"("State(s) in (\"\")"=w400) -> ("States Out"=w399:string)  [unwired: 14 in]
      }
      frame "---------- Results Data ----------" {
        # "Template Separator\n(You can make a copy of, or modify, this frame)"
        n162 = call <vilib>:"Add State(s) to Queue__jki_lib_state_machine.vi"("State(s) in (\"\")"=w404) -> ("States Out"=w403:string)  [unwired: 14 in]
      }
      frame "Results Data: Write Results Data" {
        w406 = ","  # delimiter (\t)
        w407 = TRUE  # append to file? (new file:F)
        n163 = Unbundle By Name(w409) -> ("Results File Path"=w408:path, "Results Data Array"=w405:string[][])
        "Results Data Array" <- w405
        n164 = call-poly <vilib>:"Write Delimited Spreadsheet.vi"("file path (dialog if empty)"=w408, "2D data"=w405, "append to file? (new file:F)"=w407, "error in (no error)"=w410, "delimiter (\\t)"=w406) -> ("error out"=w411:errorcluster)  [unwired: 9 in, 1 out]
        n165 = call <vilib>:"Add State(s) to Queue__jki_lib_state_machine.vi"("State(s) in (\"\")"=w413) -> ("States Out"=w412:string)  [unwired: 14 in]
      }
      frame "---------- Fuse Test ----------" {
        # "Template Separator\n(You can make a copy of, or modify, this frame)"
        n166 = call <vilib>:"Add State(s) to Queue__jki_lib_state_machine.vi"("State(s) in (\"\")"=w417) -> ("States Out"=w416:string)  [unwired: 14 in]
      }
      frame "Fuse Test: Initialise" {
        # "Get data from FGV"
        # "Measurement initialisation code goes here"
        n167 = call "FGV - Initialise.vi"("Enum"=FGV_-_Enum."Get Data", "Error In"=w422) -> ("connection ID"=w419:refnum<k16>, "Handle Out"=w418:u64, "Error Out"=w421:errorcluster)  [unwired: 10 in, 1 out]
        n168 = Bundle By Name(cluster=w424, "connection ID"=w419, "handle out"=w418) -> (w423:T5)
        n169 = call <vilib>:"Add State(s) to Queue__jki_lib_state_machine.vi"("State(s) in (\"\")"=w426) -> ("States Out"=w425:string)  [unwired: 14 in]
      }
      frame "Fuse Test: F1 Start Timer" {
        # "Template Separator\n(You can make a copy of, or modify, this frame)"
        n170 = call "Timer.vi"("error in (no error)"=w428, "Enum"=T4."Start Timer") -> ("error out"=w427:errorcluster)  [unwired: 6 in, 3 out]
        n171 = call <vilib>:"Add State(s) to Queue__jki_lib_state_machine.vi"("State(s) in (\"\")"=w432) -> ("States Out"=w431:string)  [unwired: 14 in]
      }
      frame "Fuse Test: F1 I2C Measurment" {
        # "Turn Fuse 1 Read"
        n172 = Unbundle By Name(w440) -> ("handle out"=w435:u64)
        n173 = call "PCA9525 - CJB.vi"("error in (no error)"=w436, "buffer"=u8[] [2, 254, 21], "handle"=w435) -> ("error out"=w437:errorcluster, "handle out"=w434:u64)  [unwired: 7 in]
        n174 = Bundle By Name(cluster=w440, "handle out"=w434) -> (w439:T5)
        n175 = call <vilib>:"Add State(s) to Queue__jki_lib_state_machine.vi"("State(s) in Front (\"\")"="Fuse Test: F1 UDP Read" ("State(s) in Front (\"\")"), "State(s) in (\"\")"=w442) -> ("States Out"=w441:string)  [unwired: 13 in]
      }
      frame "Fuse Test: F1 UDP Read" {
        # "Error 56 is ignored becasue it means\nUDP is blank."
        # "Change data to an array"
        # "Extract the fuse data\n from the telemetary"
        # "Read Telemetary Data"
        n176 = Unbundle By Name(w448) -> ("connection ID"=w458:refnum<k16>)
        n177 = UDP Read(connection ID=w458, timeout ms (25000)=10, 8:w449) -> (data out=w443:string, error out=w447:errorcluster, 3:w457:refnum<k16>)  [unwired: 1 in, 2 out]
        n178 = String Subset(string=w443, offset (0)=91 ("offset (0) 2"), length (rest)=1 ("length (rest) 2")) -> (substring=w456:string)
        n179 = String To Byte Array(string=w456) -> (unsigned byte array=w465:u8[])
        n180 = Equal?(x=w456, y="Â") -> (x = y?=→"Fuse 1 Test":bool)
        n181 = Number To Hexadecimal String(2:w465) -> (0:w464:string[])  [unwired: 1 in]
        n182 = Index Array(array=w464, index=0) -> (element=w451:string)
        n183 = Equal?(x=w451, y="F1") -> (x = y?=w453:bool)
        n184 = Bundle By Name(cluster=w448, "connection ID"=w457, "Fuse 1 Test"=w451) -> (w466:T5)
        n185 = call <vilib>:"Clear Errors.vi"("error in (no error)"=w447, "specific error code to clear (0: all)"=56) -> ("error out"=w446:errorcluster)  [unwired: 4 in, 1 out]
        n186 = call-poly <vilib>:"Select State(s)__jki_lib_state_machine.vi"("State(s) if True (\"\")"="Fuse Test: F2 Start Timer" ("State(s) if True (\"\")"), "Select"=w453, "State(s) if False (\"\")"="Fuse Test: F1 Elapsed Timer" ("State(s) if False (\"\")")) -> ("States Out"=w450:string)  [unwired: 12 in]
        n187 = call <vilib>:"Add State(s) to Queue__jki_lib_state_machine.vi"("State(s) in Front (\"\")"=w450, "State(s) in (\"\")"=w468) -> ("States Out"=w467:string)  [unwired: 13 in]
      }
      frame "Fuse Test: F1 Elapsed Timer" {
        # "Template Separator\n(You can make a copy of, or modify, this frame)"
        n188 = call "Timer.vi"("error in (no error)"=w472, "Target Time"=2.0, "Enum"=T4."Get Time") -> ("error out"=w471:errorcluster, "Time Elapsed?"=w473:bool)  [unwired: 5 in, 2 out]
        n189 = call-poly <vilib>:"Select State(s)__jki_lib_state_machine.vi"("State(s) if True (\"\")"="Fuse Test: F2 Start Timer" ("State(s) if True (\"\")"), "Select"=w473, "State(s) if False (\"\")"="Fuse Test: F1 UDP Read" ("State(s) if False (\"\")")) -> ("States Out"=w470:string)  [unwired: 12 in]
        n190 = call <vilib>:"Add State(s) to Queue__jki_lib_state_machine.vi"("State(s) in Front (\"\")"=w470, "State(s) in (\"\")"=w479) -> ("States Out"=w478:string)  [unwired: 13 in]
      }
      frame "Fuse Test: F2 Start Timer" {
        # "Template Separator\n(You can make a copy of, or modify, this frame)"
        n191 = call "Timer.vi"("error in (no error)"=w482, "Enum"=T4."Start Timer") -> ("error out"=w481:errorcluster)  [unwired: 6 in, 3 out]
        n192 = call <vilib>:"Add State(s) to Queue__jki_lib_state_machine.vi"("State(s) in Front (\"\")"="Fuse Test: F2 I2C Measurment" ("State(s) in Front (\"\")"), "State(s) in (\"\")"=w486) -> ("States Out"=w485:string)  [unwired: 13 in]
      }
      frame "Fuse Test: F2 I2C Measurment" {
        n193 = Unbundle By Name(w494) -> ("handle out"=w489:u64)
        n194 = call "PCA9525 - CJB.vi"("error in (no error)"=w490, "buffer"=u8[] [2, 253, 21], "handle"=w489) -> ("error out"=w491:errorcluster, "handle out"=w488:u64)  [unwired: 7 in]
        n195 = Bundle By Name(cluster=w494, "handle out"=w488) -> (w493:T5)
        n196 = call <vilib>:"Add State(s) to Queue__jki_lib_state_machine.vi"("State(s) in Front (\"\")"="Fuse Test: F2 UDP Read" ("State(s) in Front (\"\")"), "State(s) in (\"\")"=w496) -> ("States Out"=w495:string)  [unwired: 13 in]
      }
      frame "Fuse Test: F2 UDP Read" {
        # "Error 56 is ignored becasue it means\nUDP is blank."
        # "Change data to an array"
        # "Extract the fuse data\n from the telemetary"
        # "Read Telemetary Data"
        n197 = Unbundle By Name(w502) -> ("connection ID"=w512:refnum<k16>)
        n198 = UDP Read(connection ID=w512, timeout ms (25000)=100, 8:w503) -> (data out=w497:string, error out=w501:errorcluster, 3:w511:refnum<k16>)  [unwired: 1 in, 2 out]
        n199 = String Subset(string=w497, offset (0)=91 ("offset (0) 2"), length (rest)=1 ("length (rest) 2")) -> (substring=w510:string)
        n200 = String To Byte Array(string=w510) -> (unsigned byte array=w519:u8[])
        n201 = Equal?(x=w510, y="Â") -> (x = y?=→"Fuse 2 Test":bool)
        n202 = Number To Hexadecimal String(2:w519) -> (0:w518:string[])  [unwired: 1 in]
        n203 = Index Array(array=w518, index=0) -> (element=w505:string)
        n204 = Bundle By Name(cluster=w502, "connection ID"=w511, "Fuse 2 Test"=w505) -> (w520:T5)
        n205 = Equal?(x=w505, y="F1") -> (x = y?=w507:bool)
        n206 = call <vilib>:"Clear Errors.vi"("error in (no error)"=w501, "specific error code to clear (0: all)"=56) -> ("error out"=w500:errorcluster)  [unwired: 4 in, 1 out]
        n207 = call-poly <vilib>:"Select State(s)__jki_lib_state_machine.vi"("State(s) if True (\"\")"="Fuse Test: F3 Start Timer" ("State(s) if True (\"\")"), "Select"=w507, "State(s) if False (\"\")"="Fuse Test: F2 Elapsed Timer" ("State(s) if False (\"\")")) -> ("States Out"=w504:string)  [unwired: 12 in]
        n208 = call <vilib>:"Add State(s) to Queue__jki_lib_state_machine.vi"("State(s) in Front (\"\")"=w504, "State(s) in (\"\")"=w522) -> ("States Out"=w521:string)  [unwired: 13 in]
      }
      frame "Fuse Test: F2 Elapsed Timer" {
        # "Template Separator\n(You can make a copy of, or modify, this frame)"
        n209 = call "Timer.vi"("error in (no error)"=w526, "Target Time"=2.0, "Enum"=T4."Get Time") -> ("error out"=w525:errorcluster, "Time Elapsed?"=w527:bool)  [unwired: 5 in, 2 out]
        n210 = call-poly <vilib>:"Select State(s)__jki_lib_state_machine.vi"("State(s) if True (\"\")"="Fuse Test: F3 Start Timer" ("State(s) if True (\"\")"), "Select"=w527, "State(s) if False (\"\")"="Fuse Test: F2 UDP Read" ("State(s) if False (\"\")")) -> ("States Out"=w524:string)  [unwired: 12 in]
        n211 = call <vilib>:"Add State(s) to Queue__jki_lib_state_machine.vi"("State(s) in Front (\"\")"=w524, "State(s) in (\"\")"=w533) -> ("States Out"=w532:string)  [unwired: 13 in]
      }
      frame "Fuse Test: F3 Start Timer" {
        # "Template Separator\n(You can make a copy of, or modify, this frame)"
        n212 = call "Timer.vi"("error in (no error)"=w536, "Enum"=T4."Start Timer") -> ("error out"=w535:errorcluster)  [unwired: 6 in, 3 out]
        n213 = call <vilib>:"Add State(s) to Queue__jki_lib_state_machine.vi"("State(s) in Front (\"\")"="Fuse Test: F3 I2C Measurment" ("State(s) in Front (\"\")"), "State(s) in (\"\")"=w540) -> ("States Out"=w539:string)  [unwired: 13 in]
      }
      frame "Fuse Test: F3 I2C Measurment" {
        n214 = Unbundle By Name(w548) -> ("handle out"=w543:u64)
        n215 = call "PCA9525 - CJB.vi"("error in (no error)"=w544, "buffer"=u8[] [2, 254, 21], "handle"=w543) -> ("error out"=w545:errorcluster, "handle out"=w542:u64)  [unwired: 7 in]
        n216 = Bundle By Name(cluster=w548, "handle out"=w542) -> (w547:T5)
        n217 = call <vilib>:"Add State(s) to Queue__jki_lib_state_machine.vi"("State(s) in Front (\"\")"="Fuse Test: F3 UDP Read" ("State(s) in Front (\"\")"), "State(s) in (\"\")"=w550) -> ("States Out"=w549:string)  [unwired: 13 in]
      }
      frame "Fuse Test: F3 UDP Read" {
        # "Error 56 is ignored becasue it means\nUDP is blank."
        # "Change data to an array"
        # "Extract the fuse data\n from the telemetary"
        # "Read Telemetary Data"
        n218 = Unbundle By Name(w556) -> ("connection ID"=w566:refnum<k16>)
        n219 = UDP Read(connection ID=w566, timeout ms (25000)=100, 8:w557) -> (data out=w551:string, error out=w555:errorcluster, 3:w565:refnum<k16>)  [unwired: 1 in, 2 out]
        n220 = String Subset(string=w551, offset (0)=91 ("offset (0) 2"), length (rest)=1 ("length (rest) 2")) -> (substring=w564:string)
        n221 = String To Byte Array(string=w564) -> (unsigned byte array=w573:u8[])
        n222 = Equal?(x=w564, y="Â") -> (x = y?=→"Fuse 3 Test":bool)
        n223 = Number To Hexadecimal String(2:w573) -> (0:w572:string[])  [unwired: 1 in]
        n224 = Index Array(array=w572, index=0) -> (element=w559:string)
        n225 = Equal?(x=w559, y="F1") -> (x = y?=w561:bool)
        n226 = Bundle By Name(cluster=w556, "connection ID"=w565, "Fuse 3 Test"=w559) -> (w574:T5)
        n227 = call <vilib>:"Clear Errors.vi"("error in (no error)"=w555, "specific error code to clear (0: all)"=56) -> ("error out"=w554:errorcluster)  [unwired: 4 in, 1 out]
        n228 = call-poly <vilib>:"Select State(s)__jki_lib_state_machine.vi"("State(s) if True (\"\")"="Fuse Test: F4 Start Timer" ("State(s) if True (\"\")"), "Select"=w561, "State(s) if False (\"\")"="Fuse Test: F3 Elapsed Timer" ("State(s) if False (\"\")")) -> ("States Out"=w558:string)  [unwired: 12 in]
        n229 = call <vilib>:"Add State(s) to Queue__jki_lib_state_machine.vi"("State(s) in Front (\"\")"=w558, "State(s) in (\"\")"=w576) -> ("States Out"=w575:string)  [unwired: 13 in]
      }
      frame "Fuse Test: F3 Elapsed Timer" {
        # "Template Separator\n(You can make a copy of, or modify, this frame)"
        n230 = call "Timer.vi"("error in (no error)"=w580, "Target Time"=2.0, "Enum"=T4."Get Time") -> ("error out"=w579:errorcluster, "Time Elapsed?"=w581:bool)  [unwired: 5 in, 2 out]
        n231 = call-poly <vilib>:"Select State(s)__jki_lib_state_machine.vi"("State(s) if True (\"\")"="Fuse Test: F4 Start Timer" ("State(s) if True (\"\")"), "Select"=w581, "State(s) if False (\"\")"="Fuse Test: F3 UDP Read" ("State(s) if False (\"\")")) -> ("States Out"=w578:string)  [unwired: 12 in]
        n232 = call <vilib>:"Add State(s) to Queue__jki_lib_state_machine.vi"("State(s) in Front (\"\")"=w578, "State(s) in (\"\")"=w587) -> ("States Out"=w586:string)  [unwired: 13 in]
      }
      frame "Fuse Test: F4 Start Timer" {
        # "Template Separator\n(You can make a copy of, or modify, this frame)"
        n233 = call "Timer.vi"("error in (no error)"=w590, "Enum"=T4."Start Timer") -> ("error out"=w589:errorcluster)  [unwired: 6 in, 3 out]
        n234 = call <vilib>:"Add State(s) to Queue__jki_lib_state_machine.vi"("State(s) in Front (\"\")"="Fuse Test: F4 I2C Measurment" ("State(s) in Front (\"\")"), "State(s) in (\"\")"=w594) -> ("States Out"=w593:string)  [unwired: 13 in]
      }
      frame "Fuse Test: F4 I2C Measurment" {
        n235 = Unbundle By Name(w602) -> ("handle out"=w597:u64)
        n236 = call "PCA9525 - CJB.vi"("error in (no error)"=w598, "buffer"=u8[] [2, 247, 21], "handle"=w597) -> ("error out"=w599:errorcluster, "handle out"=w596:u64)  [unwired: 7 in]
        n237 = Bundle By Name(cluster=w602, "handle out"=w596) -> (w601:T5)
        n238 = call <vilib>:"Add State(s) to Queue__jki_lib_state_machine.vi"("State(s) in Front (\"\")"="Fuse Test: F4 UDP Read" ("State(s) in Front (\"\")"), "State(s) in (\"\")"=w604) -> ("States Out"=w603:string)  [unwired: 13 in]
      }
      frame "Fuse Test: F4 UDP Read" {
        # "Error 56 is ignored becasue it means\nUDP is blank."
        # "Change data to an array"
        # "Extract the fuse data\n from the telemetary"
        # "Read Telemetary Data"
        n239 = Unbundle By Name(w610) -> ("connection ID"=w620:refnum<k16>)
        n240 = UDP Read(connection ID=w620, timeout ms (25000)=100, 8:w611) -> (data out=w605:string, error out=w609:errorcluster, 3:w619:refnum<k16>)  [unwired: 1 in, 2 out]
        n241 = String Subset(string=w605, offset (0)=91 ("offset (0) 2"), length (rest)=1 ("length (rest) 2")) -> (substring=w618:string)
        n242 = String To Byte Array(string=w618) -> (unsigned byte array=w627:u8[])
        n243 = Equal?(x=w618, y="Â") -> (x = y?=→"Fuse 4 Test":bool)
        n244 = Number To Hexadecimal String(2:w627) -> (0:w626:string[])  [unwired: 1 in]
        n245 = Index Array(array=w626, index=0) -> (element=w613:string)
        n246 = Equal?(x=w613, y="F1") -> (x = y?=w615:bool)
        n247 = Bundle By Name(cluster=w610, "connection ID"=w619, "Fuse 4 Test"=w613) -> (w628:T5)
        n248 = call <vilib>:"Clear Errors.vi"("error in (no error)"=w609, "specific error code to clear (0: all)"=56) -> ("error out"=w608:errorcluster)  [unwired: 4 in, 1 out]
        n249 = call-poly <vilib>:"Select State(s)__jki_lib_state_machine.vi"("State(s) if True (\"\")"="Fuse Test: F5 Start Timer" ("State(s) if True (\"\")"), "Select"=w615, "State(s) if False (\"\")"="Fuse Test: F4 Elapsed Timer" ("State(s) if False (\"\")")) -> ("States Out"=w612:string)  [unwired: 12 in]
        n250 = call <vilib>:"Add State(s) to Queue__jki_lib_state_machine.vi"("State(s) in Front (\"\")"=w612, "State(s) in (\"\")"=w630) -> ("States Out"=w629:string)  [unwired: 13 in]
      }
      frame "Fuse Test: F4 Elapsed Timer" {
        # "Template Separator\n(You can make a copy of, or modify, this frame)"
        n251 = call "Timer.vi"("error in (no error)"=w634, "Target Time"=2.0, "Enum"=T4."Get Time") -> ("error out"=w633:errorcluster, "Time Elapsed?"=w635:bool)  [unwired: 5 in, 2 out]
        n252 = call-poly <vilib>:"Select State(s)__jki_lib_state_machine.vi"("State(s) if True (\"\")"="Fuse Test: F5 Start Timer" ("State(s) if True (\"\")"), "Select"=w635, "State(s) if False (\"\")"="Fuse Test: F4 UDP Read" ("State(s) if False (\"\")")) -> ("States Out"=w632:string)  [unwired: 12 in]
        n253 = call <vilib>:"Add State(s) to Queue__jki_lib_state_machine.vi"("State(s) in Front (\"\")"=w632, "State(s) in (\"\")"=w641) -> ("States Out"=w640:string)  [unwired: 13 in]
      }
      frame "Fuse Test: F5 Start Timer" {
        # "Template Separator\n(You can make a copy of, or modify, this frame)"
        n254 = call "Timer.vi"("error in (no error)"=w644, "Enum"=T4."Start Timer") -> ("error out"=w643:errorcluster)  [unwired: 6 in, 3 out]
        n255 = call <vilib>:"Add State(s) to Queue__jki_lib_state_machine.vi"("State(s) in Front (\"\")"="Fuse Test: F5 I2C Measurment" ("State(s) in Front (\"\")"), "State(s) in (\"\")"=w648) -> ("States Out"=w647:string)  [unwired: 13 in]
      }
      frame "Fuse Test: F5 I2C Measurment" {
        n256 = Unbundle By Name(w656) -> ("handle out"=w651:u64)
        n257 = call "PCA9525 - CJB.vi"("error in (no error)"=w652, "buffer"=u8[] [2, 239, 21], "handle"=w651) -> ("error out"=w653:errorcluster, "handle out"=w650:u64)  [unwired: 7 in]
        n258 = Bundle By Name(cluster=w656, "handle out"=w650) -> (w655:T5)
        n259 = call <vilib>:"Add State(s) to Queue__jki_lib_state_machine.vi"("State(s) in Front (\"\")"="Fuse Test: F5 UDP Read" ("State(s) in Front (\"\")"), "State(s) in (\"\")"=w658) -> ("States Out"=w657:string)  [unwired: 13 in]
      }
      frame "Fuse Test: F5 UDP Read" {
        # "Error 56 is ignored becasue it means\nUDP is blank."
        # "Change data to an array"
        # "Extract the fuse data\n from the telemetary"
        # "Read Telemetary Data"
        n260 = Unbundle By Name(w664) -> ("connection ID"=w674:refnum<k16>)
        n261 = UDP Read(connection ID=w674, timeout ms (25000)=100, 8:w665) -> (data out=w659:string, error out=w663:errorcluster, 3:w673:refnum<k16>)  [unwired: 1 in, 2 out]
        n262 = String Subset(string=w659, offset (0)=91 ("offset (0) 2"), length (rest)=1 ("length (rest) 2")) -> (substring=w672:string)
        n263 = String To Byte Array(string=w672) -> (unsigned byte array=w681:u8[])
        n264 = Equal?(x=w672, y="Â") -> (x = y?=→"Fuse 5 Test":bool)
        n265 = Number To Hexadecimal String(2:w681) -> (0:w680:string[])  [unwired: 1 in]
        n266 = Index Array(array=w680, index=0) -> (element=w667:string)
        n267 = Equal?(x=w667, y="F1") -> (x = y?=w669:bool)
        n268 = Bundle By Name(cluster=w664, "connection ID"=w673, "Fuse 5 Test"=w667) -> (w682:T5)
        n269 = call <vilib>:"Clear Errors.vi"("error in (no error)"=w663, "specific error code to clear (0: all)"=56) -> ("error out"=w662:errorcluster)  [unwired: 4 in, 1 out]
        n270 = call-poly <vilib>:"Select State(s)__jki_lib_state_machine.vi"("State(s) if True (\"\")"="Fuse Test: F6 Start Timer" ("State(s) if True (\"\")"), "Select"=w669, "State(s) if False (\"\")"="Fuse Test: F5 Elapsed Timer" ("State(s) if False (\"\")")) -> ("States Out"=w666:string)  [unwired: 12 in]
        n271 = call <vilib>:"Add State(s) to Queue__jki_lib_state_machine.vi"("State(s) in Front (\"\")"=w666, "State(s) in (\"\")"=w684) -> ("States Out"=w683:string)  [unwired: 13 in]
      }
      frame "Fuse Test: F5 Elapsed Timer" {
        # "Template Separator\n(You can make a copy of, or modify, this frame)"
        n272 = call "Timer.vi"("error in (no error)"=w688, "Target Time"=2.0, "Enum"=T4."Get Time") -> ("error out"=w687:errorcluster, "Time Elapsed?"=w689:bool)  [unwired: 5 in, 2 out]
        n273 = call-poly <vilib>:"Select State(s)__jki_lib_state_machine.vi"("State(s) if True (\"\")"="Fuse Test: F6 Start Timer" ("State(s) if True (\"\")"), "Select"=w689, "State(s) if False (\"\")"="Fuse Test: F5 UDP Read" ("State(s) if False (\"\")")) -> ("States Out"=w686:string)  [unwired: 12 in]
        n274 = call <vilib>:"Add State(s) to Queue__jki_lib_state_machine.vi"("State(s) in Front (\"\")"=w686, "State(s) in (\"\")"=w695) -> ("States Out"=w694:string)  [unwired: 13 in]
      }
      frame "Fuse Test: F6 Start Timer" {
        # "Template Separator\n(You can make a copy of, or modify, this frame)"
        n275 = call "Timer.vi"("error in (no error)"=w698, "Enum"=T4."Start Timer") -> ("error out"=w697:errorcluster)  [unwired: 6 in, 3 out]
        n276 = call <vilib>:"Add State(s) to Queue__jki_lib_state_machine.vi"("State(s) in Front (\"\")"="Fuse Test: F6 I2C Measurment" ("State(s) in Front (\"\")"), "State(s) in (\"\")"=w702) -> ("States Out"=w701:string)  [unwired: 13 in]
      }
      frame "Fuse Test: F6 I2C Measurment" {
        n277 = Unbundle By Name(w710) -> ("handle out"=w705:u64)
        n278 = call "PCA9525 - CJB.vi"("error in (no error)"=w706, "buffer"=u8[] [2, 223, 21], "handle"=w705) -> ("error out"=w707:errorcluster, "handle out"=w704:u64)  [unwired: 7 in]
        n279 = Bundle By Name(cluster=w710, "handle out"=w704) -> (w709:T5)
        n280 = call <vilib>:"Add State(s) to Queue__jki_lib_state_machine.vi"("State(s) in Front (\"\")"="Fuse Test: F6 UDP Read" ("State(s) in Front (\"\")"), "State(s) in (\"\")"=w712) -> ("States Out"=w711:string)  [unwired: 13 in]
      }
      frame "Fuse Test: F6 UDP Read" {
        # "Error 56 is ignored becasue it means\nUDP is blank."
        # "Change data to an array"
        # "Extract the fuse data\n from the telemetary"
        # "Read Telemetary Data"
        n281 = Unbundle By Name(w718) -> ("connection ID"=w728:refnum<k16>)
        n282 = UDP Read(connection ID=w728, timeout ms (25000)=100, 8:w719) -> (data out=w713:string, error out=w717:errorcluster, 3:w727:refnum<k16>)  [unwired: 1 in, 2 out]
        n283 = String Subset(string=w713, offset (0)=91 ("offset (0) 2"), length (rest)=1 ("length (rest) 2")) -> (substring=w726:string)
        n284 = String To Byte Array(string=w726) -> (unsigned byte array=w735:u8[])
        n285 = Equal?(x=w726, y="Â") -> (x = y?=→"Fuse 6 Test":bool)
        n286 = Number To Hexadecimal String(2:w735) -> (0:w734:string[])  [unwired: 1 in]
        n287 = Index Array(array=w734, index=0) -> (element=w721:string)
        n288 = Equal?(x=w721, y="F1") -> (x = y?=w723:bool)
        n289 = Bundle By Name(cluster=w718, "connection ID"=w727, "Fuse 6 Test"=w721) -> (w736:T5)
        n290 = call <vilib>:"Clear Errors.vi"("error in (no error)"=w717, "specific error code to clear (0: all)"=56) -> ("error out"=w716:errorcluster)  [unwired: 4 in, 1 out]
        n291 = call-poly <vilib>:"Select State(s)__jki_lib_state_machine.vi"("State(s) if True (\"\")"="Fuse Test: F7 Start Timer" ("State(s) if True (\"\")"), "Select"=w723, "State(s) if False (\"\")"="Fuse Test: F6 Elapsed Timer" ("State(s) if False (\"\")")) -> ("States Out"=w720:string)  [unwired: 12 in]
        n292 = call <vilib>:"Add State(s) to Queue__jki_lib_state_machine.vi"("State(s) in Front (\"\")"=w720, "State(s) in (\"\")"=w738) -> ("States Out"=w737:string)  [unwired: 13 in]
      }
      frame "Fuse Test: F6 Elapsed Timer" {
        # "Template Separator\n(You can make a copy of, or modify, this frame)"
        n293 = call "Timer.vi"("error in (no error)"=w742, "Target Time"=2.0, "Enum"=T4."Get Time") -> ("error out"=w741:errorcluster, "Time Elapsed?"=w743:bool)  [unwired: 5 in, 2 out]
        n294 = call-poly <vilib>:"Select State(s)__jki_lib_state_machine.vi"("State(s) if True (\"\")"="Fuse Test: F7 Start Timer" ("State(s) if True (\"\")"), "Select"=w743, "State(s) if False (\"\")"="Fuse Test: F6 UDP Read" ("State(s) if False (\"\")")) -> ("States Out"=w740:string)  [unwired: 12 in]
        n295 = call <vilib>:"Add State(s) to Queue__jki_lib_state_machine.vi"("State(s) in Front (\"\")"=w740, "State(s) in (\"\")"=w749) -> ("States Out"=w748:string)  [unwired: 13 in]
      }
      frame "Fuse Test: F7 Start Timer" {
        # "Template Separator\n(You can make a copy of, or modify, this frame)"
        n296 = call "Timer.vi"("error in (no error)"=w752, "Enum"=T4."Start Timer") -> ("error out"=w751:errorcluster)  [unwired: 6 in, 3 out]
        n297 = call <vilib>:"Add State(s) to Queue__jki_lib_state_machine.vi"("State(s) in Front (\"\")"="Fuse Test: F7 I2C Measurment" ("State(s) in Front (\"\")"), "State(s) in (\"\")"=w756) -> ("States Out"=w755:string)  [unwired: 13 in]
      }
      frame "Fuse Test: F7 I2C Measurment" {
        n298 = Unbundle By Name(w764) -> ("handle out"=w759:u64)
        n299 = call "PCA9525 - CJB.vi"("error in (no error)"=w760, "buffer"=u8[] [2, 191, 21], "handle"=w759) -> ("error out"=w761:errorcluster, "handle out"=w758:u64)  [unwired: 7 in]
        n300 = Bundle By Name(cluster=w764, "handle out"=w758) -> (w763:T5)
        n301 = call <vilib>:"Add State(s) to Queue__jki_lib_state_machine.vi"("State(s) in Front (\"\")"="Fuse Test: F7 UDP Read" ("State(s) in Front (\"\")"), "State(s) in (\"\")"=w766) -> ("States Out"=w765:string)  [unwired: 13 in]
      }
      frame "Fuse Test: F7 UDP Read" {
        # "Error 56 is ignored becasue it means\nUDP is blank."
        # "Change data to an array"
        # "Extract the fuse data\n from the telemetary"
        # "Read Telemetary Data"
        n302 = Unbundle By Name(w772) -> ("connection ID"=w782:refnum<k16>)
        n303 = UDP Read(connection ID=w782, timeout ms (25000)=100, 8:w773) -> (data out=w767:string, error out=w771:errorcluster, 3:w781:refnum<k16>)  [unwired: 1 in, 2 out]
        n304 = String Subset(string=w767, offset (0)=91 ("offset (0) 2"), length (rest)=1 ("length (rest) 2")) -> (substring=w780:string)
        n305 = String To Byte Array(string=w780) -> (unsigned byte array=w789:u8[])
        n306 = Equal?(x=w780, y="Â") -> (x = y?=→"Fuse 7 Test":bool)
        n307 = Number To Hexadecimal String(2:w789) -> (0:w788:string[])  [unwired: 1 in]
        n308 = Index Array(array=w788, index=0) -> (element=w775:string)
        n309 = Equal?(x=w775, y="F1") -> (x = y?=w777:bool)
        n310 = Bundle By Name(cluster=w772, "connection ID"=w781, "Fuse 7 Test"=w775) -> (w790:T5)
        n311 = call <vilib>:"Clear Errors.vi"("error in (no error)"=w771, "specific error code to clear (0: all)"=56) -> ("error out"=w770:errorcluster)  [unwired: 4 in, 1 out]
        n312 = call-poly <vilib>:"Select State(s)__jki_lib_state_machine.vi"("State(s) if True (\"\")"="Fuse Test: F8 Start Timer" ("State(s) if True (\"\")"), "Select"=w777, "State(s) if False (\"\")"="Fuse Test: F7 Elapsed Timer" ("State(s) if False (\"\")")) -> ("States Out"=w774:string)  [unwired: 12 in]
        n313 = call <vilib>:"Add State(s) to Queue__jki_lib_state_machine.vi"("State(s) in Front (\"\")"=w774, "State(s) in (\"\")"=w792) -> ("States Out"=w791:string)  [unwired: 13 in]
      }
      frame "Fuse Test: F7 Elapsed Timer" {
        # "Template Separator\n(You can make a copy of, or modify, this frame)"
        n314 = call "Timer.vi"("error in (no error)"=w796, "Target Time"=2.0, "Enum"=T4."Get Time") -> ("error out"=w795:errorcluster, "Time Elapsed?"=w797:bool)  [unwired: 5 in, 2 out]
        n315 = call-poly <vilib>:"Select State(s)__jki_lib_state_machine.vi"("State(s) if True (\"\")"="Fuse Test: F8 Start Timer" ("State(s) if True (\"\")"), "Select"=w797, "State(s) if False (\"\")"="Fuse Test: F7 UDP Read" ("State(s) if False (\"\")")) -> ("States Out"=w794:string)  [unwired: 12 in]
        n316 = call <vilib>:"Add State(s) to Queue__jki_lib_state_machine.vi"("State(s) in Front (\"\")"=w794, "State(s) in (\"\")"=w803) -> ("States Out"=w802:string)  [unwired: 13 in]
      }
      frame "Fuse Test: F8 Start Timer" {
        # "Template Separator\n(You can make a copy of, or modify, this frame)"
        n317 = call "Timer.vi"("error in (no error)"=w806, "Enum"=T4."Start Timer") -> ("error out"=w805:errorcluster)  [unwired: 6 in, 3 out]
        n318 = call <vilib>:"Add State(s) to Queue__jki_lib_state_machine.vi"("State(s) in Front (\"\")"="Fuse Test: F8 I2C Measurment" ("State(s) in Front (\"\")"), "State(s) in (\"\")"=w810) -> ("States Out"=w809:string)  [unwired: 13 in]
      }
      frame "Fuse Test: F8 I2C Measurment" {
        n319 = Unbundle By Name(w818) -> ("handle out"=w813:u64)
        n320 = call "PCA9525 - CJB.vi"("error in (no error)"=w814, "buffer"=u8[] [2, 127, 21], "handle"=w813) -> ("error out"=w815:errorcluster, "handle out"=w812:u64)  [unwired: 7 in]
        n321 = Bundle By Name(cluster=w818, "handle out"=w812) -> (w817:T5)
        n322 = call <vilib>:"Add State(s) to Queue__jki_lib_state_machine.vi"("State(s) in Front (\"\")"="Fuse Test: F8 UDP Read" ("State(s) in Front (\"\")"), "State(s) in (\"\")"=w820) -> ("States Out"=w819:string)  [unwired: 13 in]
      }
      frame "Fuse Test: F8 UDP Read" {
        # "Error 56 is ignored becasue it means\nUDP is blank."
        # "Change data to an array"
        # "Extract the fuse data\n from the telemetary"
        # "Read Telemetary Data"
        n323 = Unbundle By Name(w826) -> ("connection ID"=w836:refnum<k16>)
        n324 = UDP Read(connection ID=w836, timeout ms (25000)=100, 8:w827) -> (data out=w821:string, error out=w825:errorcluster, 3:w835:refnum<k16>)  [unwired: 1 in, 2 out]
        n325 = String Subset(string=w821, offset (0)=91 ("offset (0) 2"), length (rest)=1 ("length (rest) 2")) -> (substring=w834:string)
        n326 = String To Byte Array(string=w834) -> (unsigned byte array=w843:u8[])
        n327 = Equal?(x=w834, y="Â") -> (x = y?=→"Fuse 8 Test":bool)
        n328 = Number To Hexadecimal String(2:w843) -> (0:w842:string[])  [unwired: 1 in]
        n329 = Index Array(array=w842, index=0) -> (element=w829:string)
        n330 = Equal?(x=w829, y="F1") -> (x = y?=w831:bool)
        n331 = Bundle By Name(cluster=w826, "connection ID"=w835, "Fuse 8 Test"=w829) -> (w844:T5)
        n332 = call <vilib>:"Clear Errors.vi"("error in (no error)"=w825, "specific error code to clear (0: all)"=56) -> ("error out"=w824:errorcluster)  [unwired: 4 in, 1 out]
        n333 = call-poly <vilib>:"Select State(s)__jki_lib_state_machine.vi"("State(s) if True (\"\")"="Fuse Test: F9 Start Timer" ("State(s) if True (\"\")"), "Select"=w831, "State(s) if False (\"\")"="Fuse Test: F8 Elapsed Timer" ("State(s) if False (\"\")")) -> ("States Out"=w828:string)  [unwired: 12 in]
        n334 = call <vilib>:"Add State(s) to Queue__jki_lib_state_machine.vi"("State(s) in Front (\"\")"=w828, "State(s) in (\"\")"=w846) -> ("States Out"=w845:string)  [unwired: 13 in]
      }
      frame "Fuse Test: F8 Elapsed Timer" {
        # "Template Separator\n(You can make a copy of, or modify, this frame)"
        n335 = call "Timer.vi"("error in (no error)"=w850, "Target Time"=2.0, "Enum"=T4."Get Time") -> ("error out"=w849:errorcluster, "Time Elapsed?"=w851:bool)  [unwired: 5 in, 2 out]
        n336 = call-poly <vilib>:"Select State(s)__jki_lib_state_machine.vi"("State(s) if True (\"\")"="Fuse Test: F9 Start Timer" ("State(s) if True (\"\")"), "Select"=w851, "State(s) if False (\"\")"="Fuse Test: F8 UDP Read" ("State(s) if False (\"\")")) -> ("States Out"=w848:string)  [unwired: 12 in]
        n337 = call <vilib>:"Add State(s) to Queue__jki_lib_state_machine.vi"("State(s) in Front (\"\")"=w848, "State(s) in (\"\")"=w857) -> ("States Out"=w856:string)  [unwired: 13 in]
      }
      frame "Fuse Test: F9 Start Timer" {
        # "Template Separator\n(You can make a copy of, or modify, this frame)"
        n338 = call "Timer.vi"("error in (no error)"=w860, "Enum"=T4."Start Timer") -> ("error out"=w859:errorcluster)  [unwired: 6 in, 3 out]
        n339 = call <vilib>:"Add State(s) to Queue__jki_lib_state_machine.vi"("State(s) in Front (\"\")"="Fuse Test: F9 I2C Measurment" ("State(s) in Front (\"\")"), "State(s) in (\"\")"=w864) -> ("States Out"=w863:string)  [unwired: 13 in]
      }
      frame "Fuse Test: F9 I2C Measurment" {
        n340 = Unbundle By Name(w872) -> ("handle out"=w867:u64)
        n341 = call "PCA9525 - CJB.vi"("error in (no error)"=w868, "buffer"=u8[] [2, 255, 50], "handle"=w867) -> ("error out"=w869:errorcluster, "handle out"=w866:u64)  [unwired: 7 in]
        n342 = Bundle By Name(cluster=w872, "handle out"=w866) -> (w871:T5)
        n343 = call <vilib>:"Add State(s) to Queue__jki_lib_state_machine.vi"("State(s) in Front (\"\")"="Fuse Test: F9 UDP Read" ("State(s) in Front (\"\")"), "State(s) in (\"\")"=w874) -> ("States Out"=w873:string)  [unwired: 13 in]
      }
      frame "Fuse Test: F9 UDP Read" {
        # "Error 56 is ignored becasue it means\nUDP is blank."
        # "Change data to an array"
        # "Extract the fuse data\n from the telemetary"
        # "Read Telemetary Data"
        n344 = Unbundle By Name(w880) -> ("connection ID"=w890:refnum<k16>)
        n345 = UDP Read(connection ID=w890, timeout ms (25000)=100, 8:w881) -> (data out=w875:string, error out=w879:errorcluster, 3:w889:refnum<k16>)  [unwired: 1 in, 2 out]
        n346 = String Subset(string=w875, offset (0)=91 ("offset (0) 2"), length (rest)=1 ("length (rest) 2")) -> (substring=w888:string)
        n347 = String To Byte Array(string=w888) -> (unsigned byte array=w897:u8[])
        n348 = Equal?(x=w888, y="Â") -> (x = y?=→"Fuse 9 Test":bool)
        n349 = Number To Hexadecimal String(2:w897) -> (0:w896:string[])  [unwired: 1 in]
        n350 = Index Array(array=w896, index=0) -> (element=w883:string)
        n351 = Equal?(x=w883, y="F1") -> (x = y?=w885:bool)
        n352 = Bundle By Name(cluster=w880, "connection ID"=w889, "Fuse 9 Test"=w883) -> (w898:T5)
        n353 = call <vilib>:"Clear Errors.vi"("error in (no error)"=w879, "specific error code to clear (0: all)"=56) -> ("error out"=w878:errorcluster)  [unwired: 4 in, 1 out]
        n354 = call-poly <vilib>:"Select State(s)__jki_lib_state_machine.vi"("State(s) if True (\"\")"="Fuse Test: All Fuses Start Timer" ("State(s) if True (\"\")"), "Select"=w885, "State(s) if False (\"\")"="Fuse Test: F9 Elapsed Timer" ("State(s) if False (\"\")")) -> ("States Out"=w882:string)  [unwired: 12 in]
        n355 = call <vilib>:"Add State(s) to Queue__jki_lib_state_machine.vi"("State(s) in Front (\"\")"=w882, "State(s) in (\"\")"=w900) -> ("States Out"=w899:string)  [unwired: 13 in]
      }
      frame "Fuse Test: F9 Elapsed Timer" {
        # "Template Separator\n(You can make a copy of, or modify, this frame)"
        n356 = call "Timer.vi"("error in (no error)"=w904, "Target Time"=2.0, "Enum"=T4."Get Time") -> ("error out"=w903:errorcluster, "Time Elapsed?"=w905:bool)  [unwired: 5 in, 2 out]
        n357 = call-poly <vilib>:"Select State(s)__jki_lib_state_machine.vi"("State(s) if True (\"\")"="Fuse Test: All Fuses Start Timer" ("State(s) if True (\"\")"), "Select"=w905, "State(s) if False (\"\")"="Fuse Test: F9 UDP Read" ("State(s) if False (\"\")")) -> ("States Out"=w902:string)  [unwired: 12 in]
        n358 = call <vilib>:"Add State(s) to Queue__jki_lib_state_machine.vi"("State(s) in Front (\"\")"=w902, "State(s) in (\"\")"=w911) -> ("States Out"=w910:string)  [unwired: 13 in]
      }
      frame "Fuse Test: All Fuses Start Timer" {
        # "Template Separator\n(You can make a copy of, or modify, this frame)"
        n359 = call "Timer.vi"("error in (no error)"=w914, "Enum"=T4."Start Timer") -> ("error out"=w913:errorcluster)  [unwired: 6 in, 3 out]
        n360 = call <vilib>:"Add State(s) to Queue__jki_lib_state_machine.vi"("State(s) in Front (\"\")"="Fuse Test: All Fuses I2C Measurment" ("State(s) in Front (\"\")"), "State(s) in (\"\")"=w918) -> ("States Out"=w917:string)  [unwired: 13 in]
      }
      frame "Fuse Test: All Fuses I2C Measurment" {
        n361 = Unbundle By Name(w926) -> ("handle out"=w921:u64)
        n362 = call "PCA9525 - CJB.vi"("error in (no error)"=w922, "buffer"=u8[] [2, 0, 18], "handle"=w921) -> ("error out"=w923:errorcluster, "handle out"=w920:u64)  [unwired: 7 in]
        n363 = Bundle By Name(cluster=w926, "handle out"=w920) -> (w925:T5)
        n364 = call <vilib>:"Add State(s) to Queue__jki_lib_state_machine.vi"("State(s) in Front (\"\")"="Fuse Test: All Fuses UDP Read" ("State(s) in Front (\"\")"), "State(s) in (\"\")"=w928) -> ("States Out"=w927:string)  [unwired: 13 in]
      }
      frame "Fuse Test: All Fuses UDP Read" {
        # "Error 56 is ignored becasue it means\nUDP is blank."
        # "Change data to an array"
        # "Extract the fuse data\n from the telemetary"
        # "Read Telemetary Data"
        n365 = Unbundle By Name(w934) -> ("connection ID"=w944:refnum<k16>)
        n366 = UDP Read(connection ID=w944, timeout ms (25000)=100, 8:w935) -> (data out=w929:string, error out=w933:errorcluster, 3:w943:refnum<k16>)  [unwired: 1 in, 2 out]
        n367 = String Subset(string=w929, offset (0)=91 ("offset (0) 2"), length (rest)=1 ("length (rest) 2")) -> (substring=w942:string)
        n368 = String To Byte Array(string=w942) -> (unsigned byte array=w951:u8[])
        n369 = Equal?(x=w942, y="Â") -> (x = y?=→"All Fuses Test":bool)
        n370 = Number To Hexadecimal String(2:w951) -> (0:w950:string[])  [unwired: 1 in]
        n371 = Index Array(array=w950, index=0) -> (element=w937:string)
        n372 = Equal?(x=w937, y="F1") -> (x = y?=w939:bool)
        n373 = Bundle By Name(cluster=w934, "connection ID"=w943, "All Fuses Test"=w937) -> (w952:T5)
        n374 = call <vilib>:"Clear Errors.vi"("error in (no error)"=w933, "specific error code to clear (0: all)"=56) -> ("error out"=w932:errorcluster)  [unwired: 4 in, 1 out]
        n375 = call-poly <vilib>:"Select State(s)__jki_lib_state_machine.vi"("State(s) if True (\"\")"="Macro: Limits" ("State(s) if True (\"\")"), "Select"=w939, "State(s) if False (\"\")"="Fuse Test: All Fuses Elapsed Timer" ("State(s) if False (\"\")")) -> ("States Out"=w936:string)  [unwired: 12 in]
        n376 = call <vilib>:"Add State(s) to Queue__jki_lib_state_machine.vi"("State(s) in Front (\"\")"=w936, "State(s) in (\"\")"=w954) -> ("States Out"=w953:string)  [unwired: 13 in]
      }
      frame "Fuse Test: All Fuses Elapsed Timer" {
        # "Template Separator\n(You can make a copy of, or modify, this frame)"
        n377 = call "Timer.vi"("error in (no error)"=w958, "Target Time"=2.0, "Enum"=T4."Get Time") -> ("error out"=w957:errorcluster, "Time Elapsed?"=w959:bool)  [unwired: 5 in, 2 out]
        n378 = call-poly <vilib>:"Select State(s)__jki_lib_state_machine.vi"("State(s) if True (\"\")"="Macro: Limits" ("State(s) if True (\"\")"), "Select"=w959, "State(s) if False (\"\")"="Fuse Test: All Fuses UDP Read" ("State(s) if False (\"\")")) -> ("States Out"=w956:string)  [unwired: 12 in]
        n379 = call <vilib>:"Add State(s) to Queue__jki_lib_state_machine.vi"("State(s) in Front (\"\")"=w956, "State(s) in (\"\")"=w965) -> ("States Out"=w964:string)  [unwired: 13 in]
      }
      frame "Fuse Test: Cleanup" {
        # "Measurment cleanup code goes here"
        n380 = Unbundle By Name(w972) -> ("handle out"=w969:u64)
        n381 = call "PCA9525 - CJB.vi"("error in (no error)"=w966, "buffer"=u8[] [2, 255, 19], "handle"=w969) -> ("error out"=w967:errorcluster, "handle out"=w968:u64)  [unwired: 7 in]
        n382 = Bundle By Name(cluster=w972, "handle out"=w968) -> (w971:T5)
        n383 = call <vilib>:"Add State(s) to Queue__jki_lib_state_machine.vi"("State(s) in (\"\")"=w974) -> ("States Out"=w973:string)  [unwired: 14 in]
      }
    }
  }
  "error out" <- w1
